vi "myRIO_BRig_RT_dataMTrig_main__wWarmUp.vi"(0 "input_dataMTrig":u16[](array[numeric]), 2 "input_Solenoid_trig_L":bool, 3 "input_Solenoid_trig_R":bool, 4 "input_Audio_trig_L":bool, 5 "input_Audio_trig_R":bool, 7 "input_Laser_trig":bool, 8 "WarmUp":bool) -> (13 "output_Laser":bool, 14 "output_dataMTrig":u16[](array[numeric]), 16 "output_Solenoid_L":bool, 17 "output_Solenoid_R":bool, 18 "output_Audio_L":bool, 19 "output_Audio_R":bool)   [LabVIEW 2014]
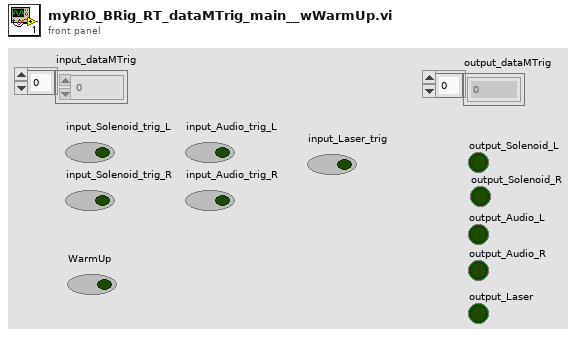
[diagram p1: front panel]
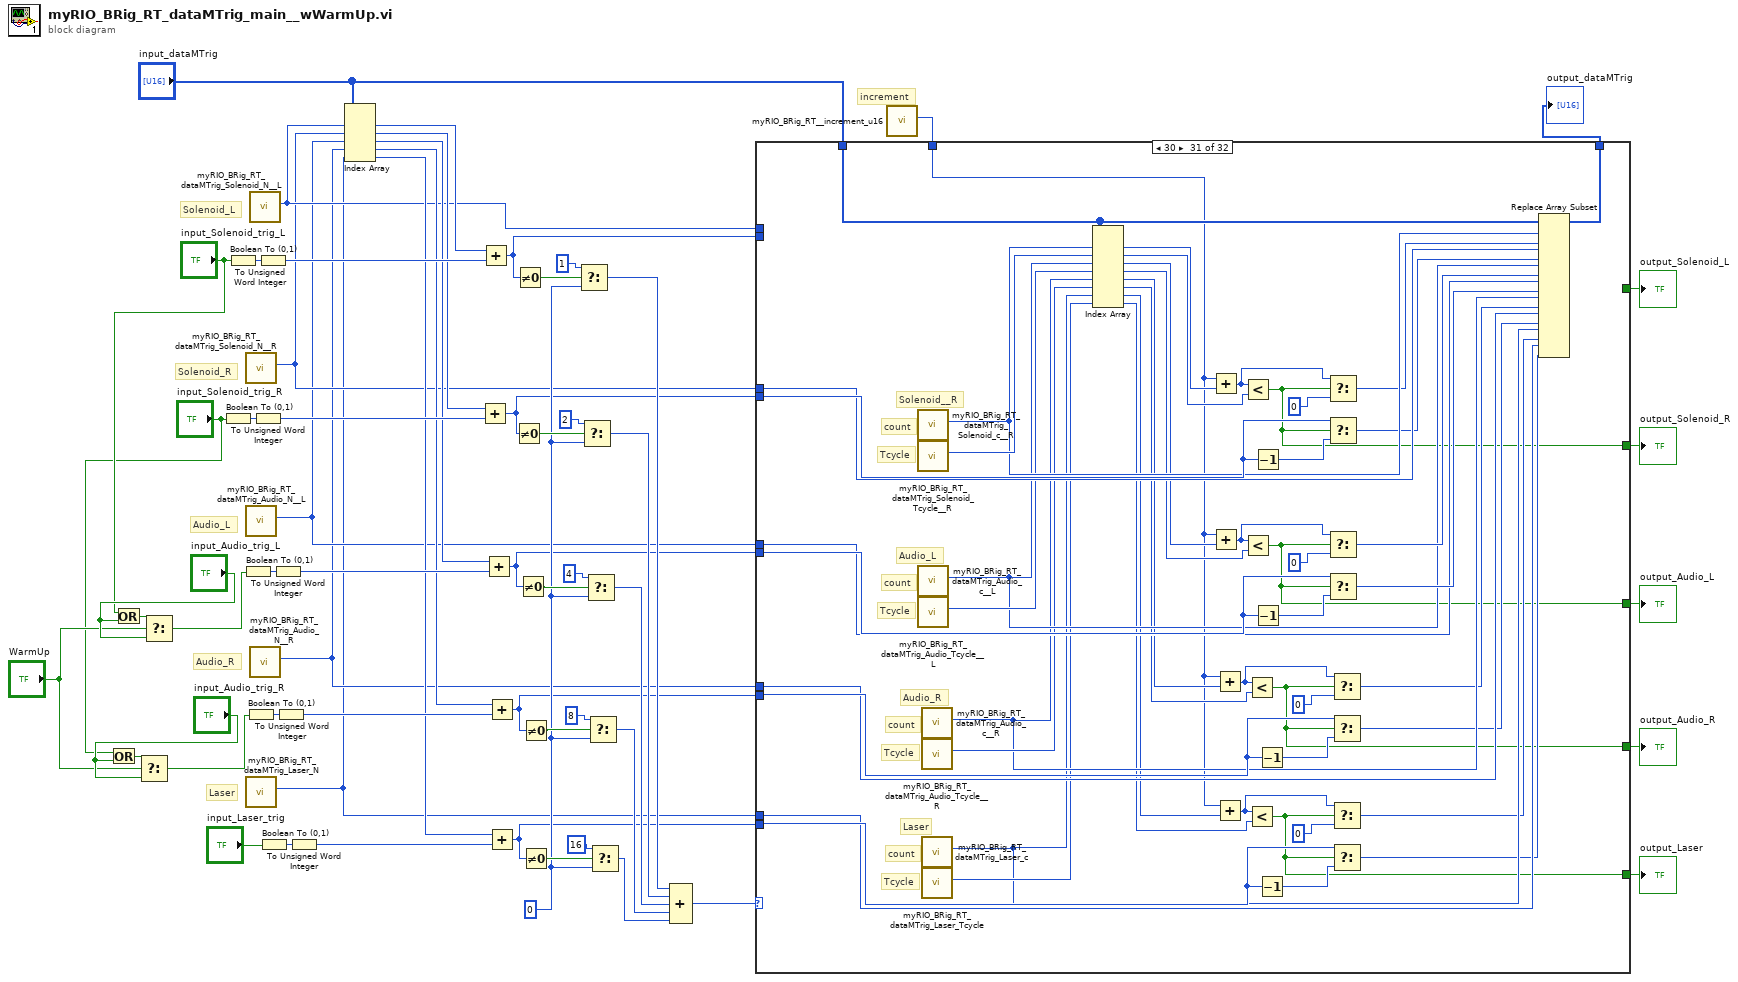
[diagram p0: block diagram]
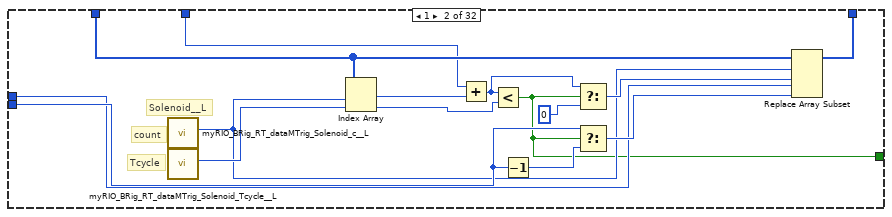
[diagram p3: hidden frame]
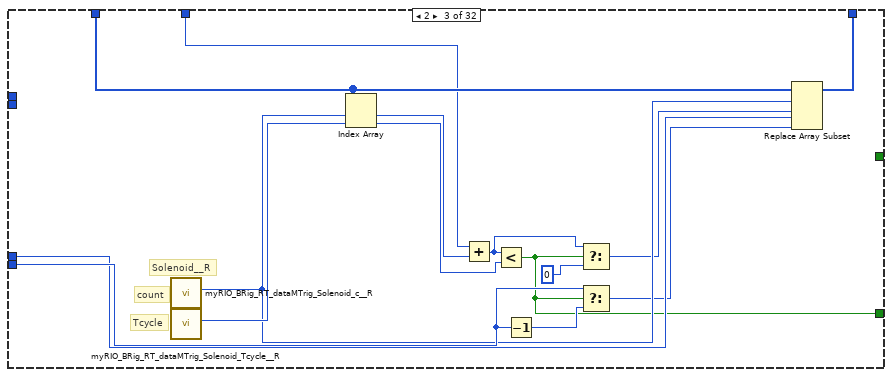
[diagram p4: hidden frame]
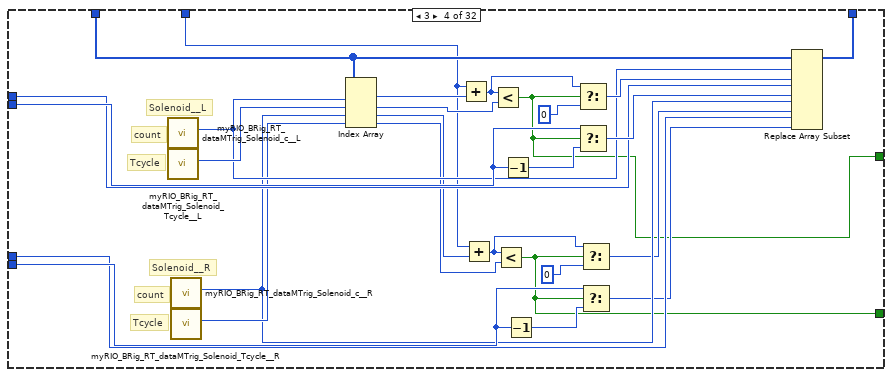
[diagram p5: hidden frame]
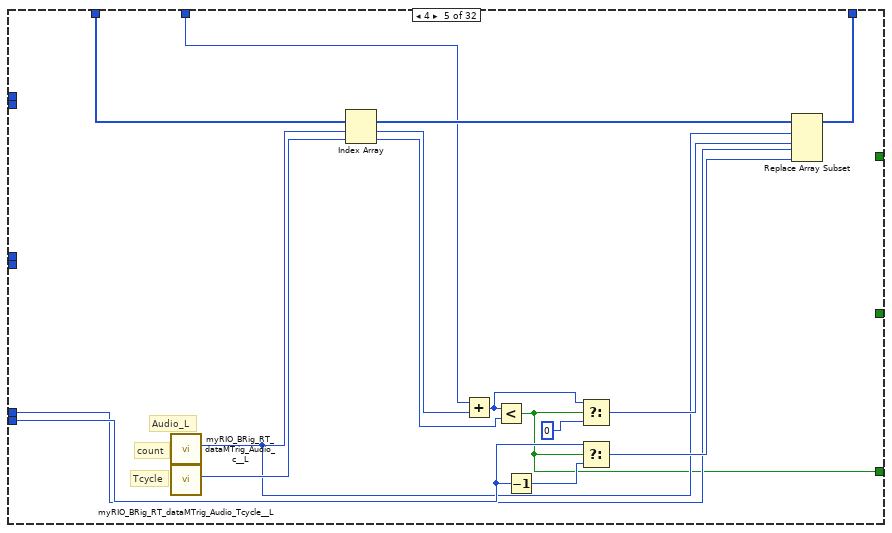
[diagram p6: hidden frame]
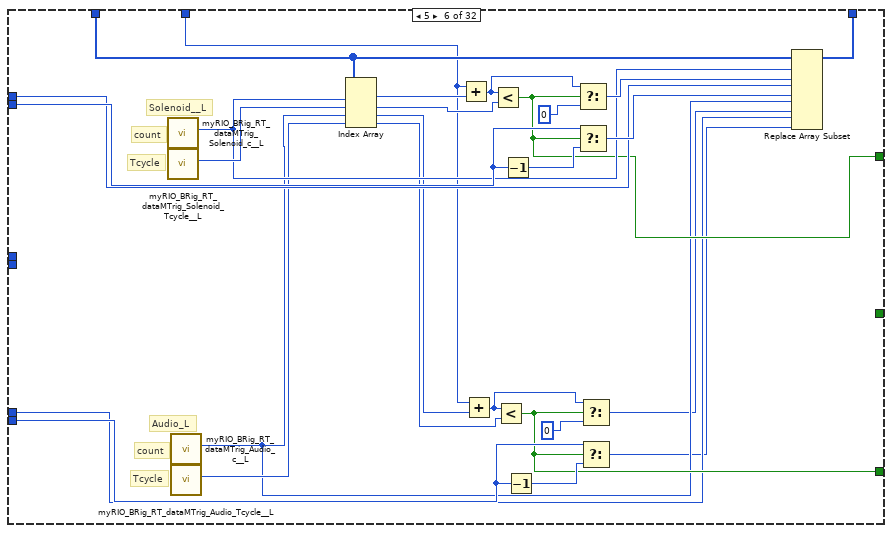
[diagram p7: hidden frame]
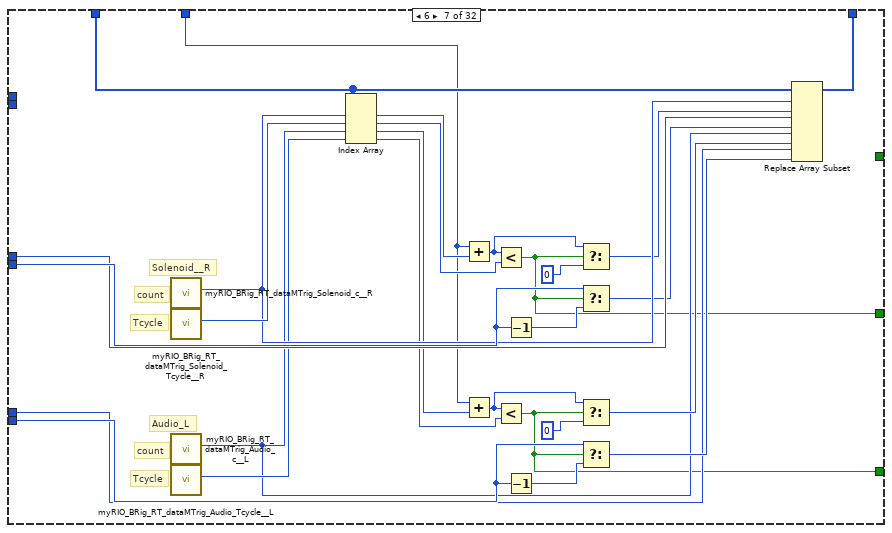
[diagram p8: hidden frame]
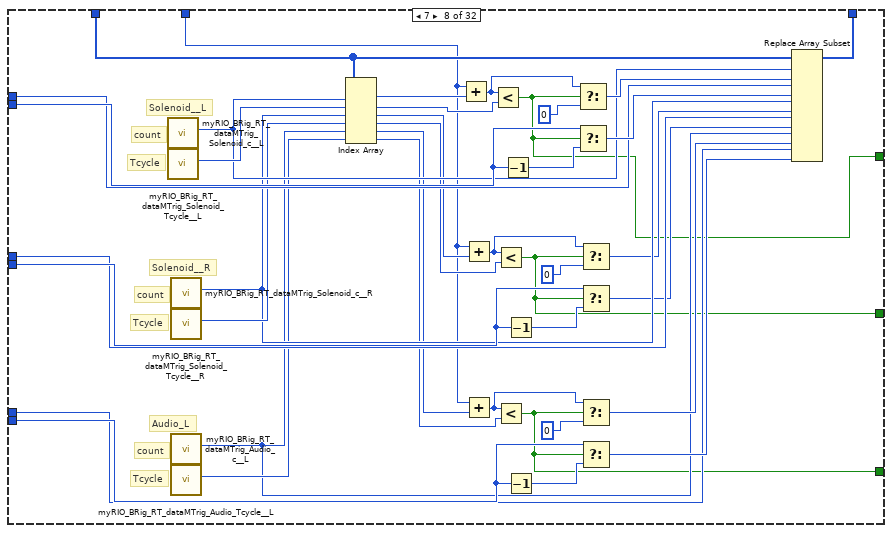
[diagram p9: hidden frame]
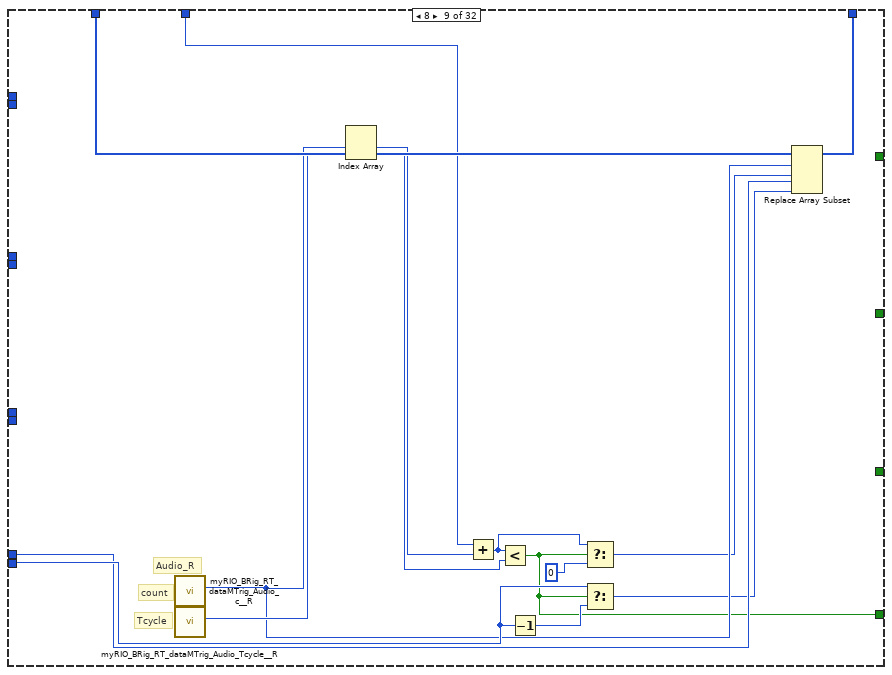
[diagram p10: hidden frame]
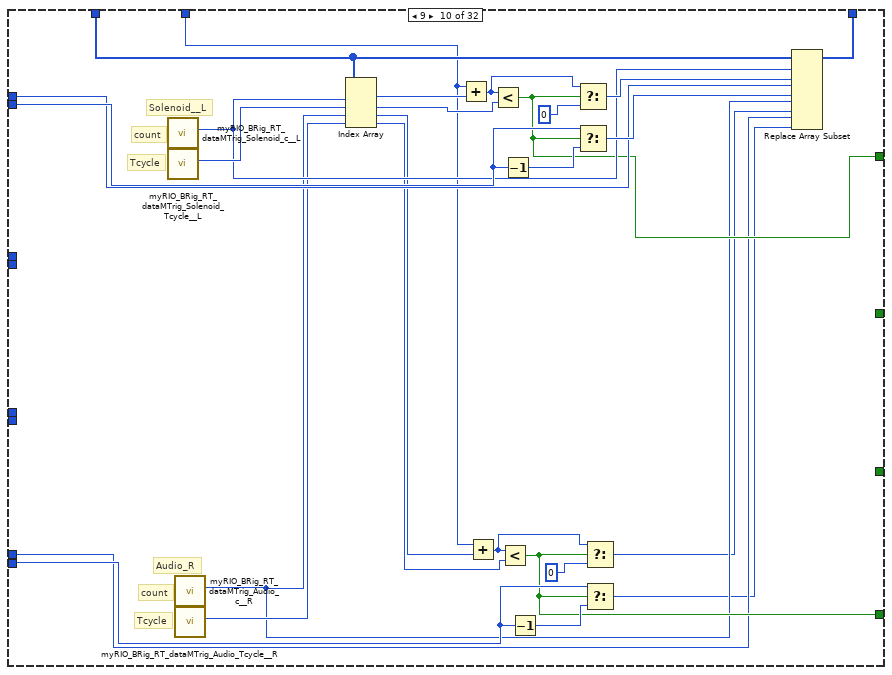
[diagram p11: hidden frame]
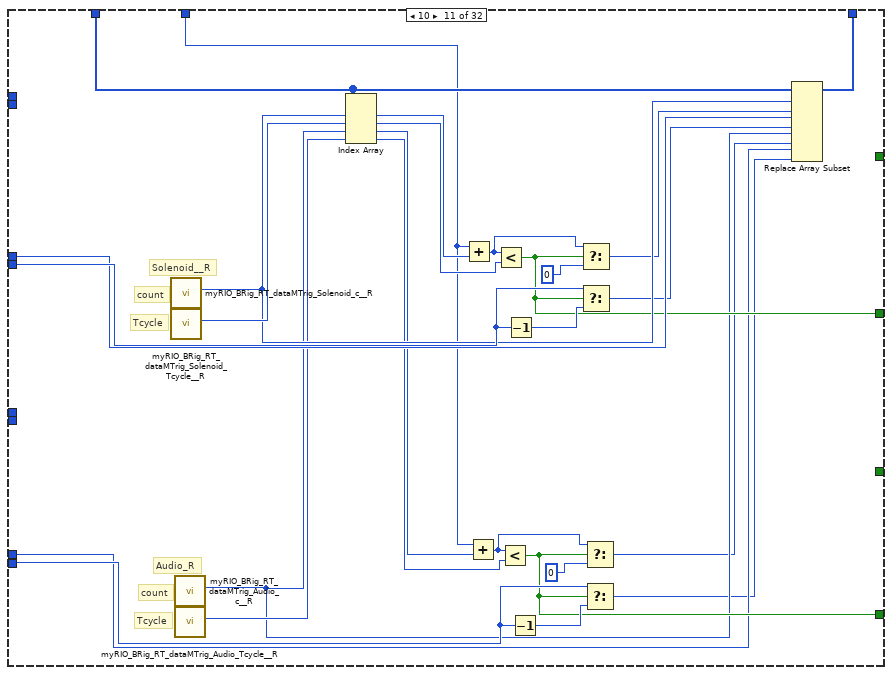
[diagram p12: hidden frame]
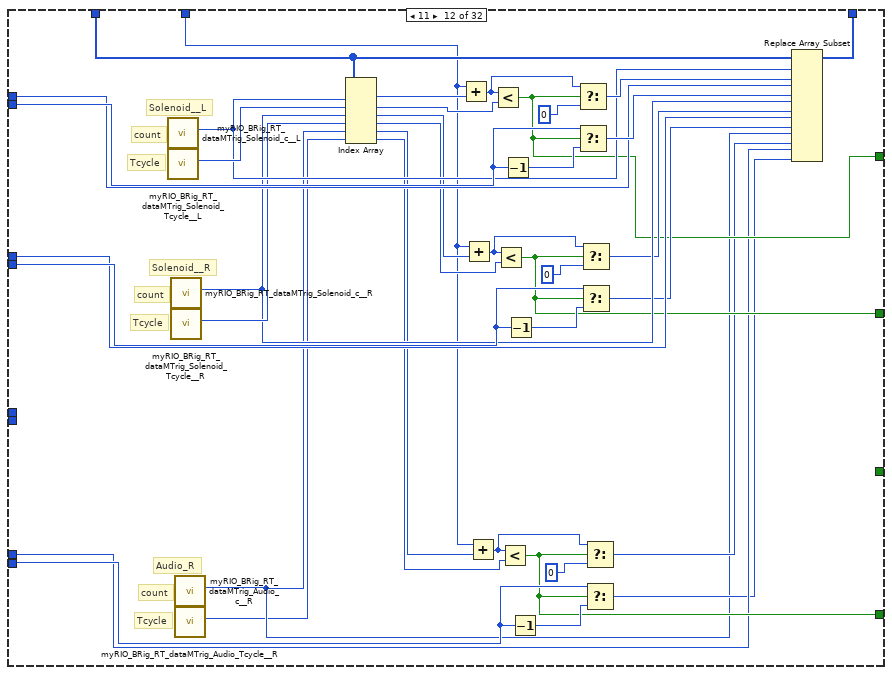
[diagram p13: hidden frame]
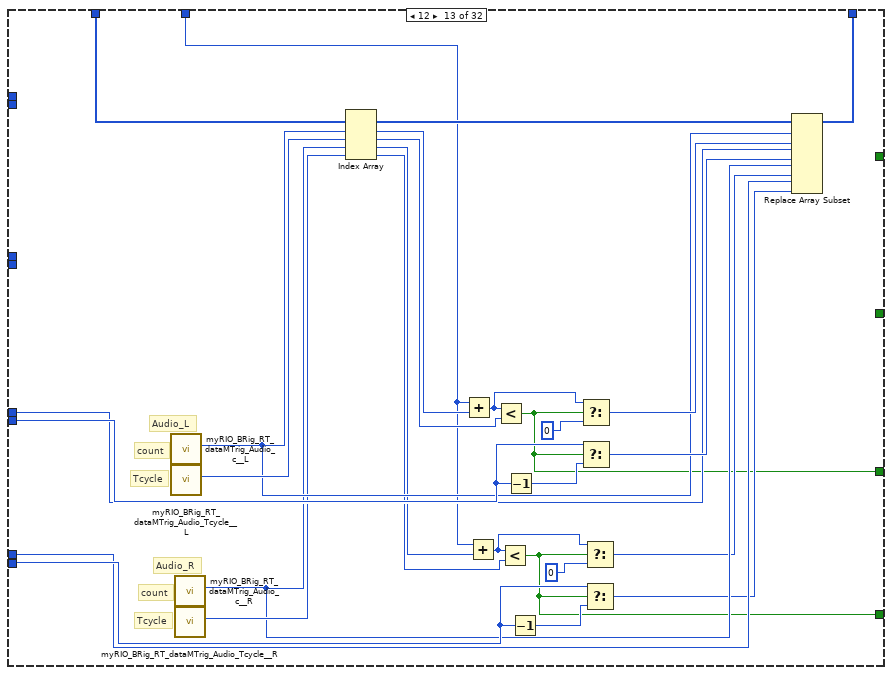
[diagram p14: hidden frame]
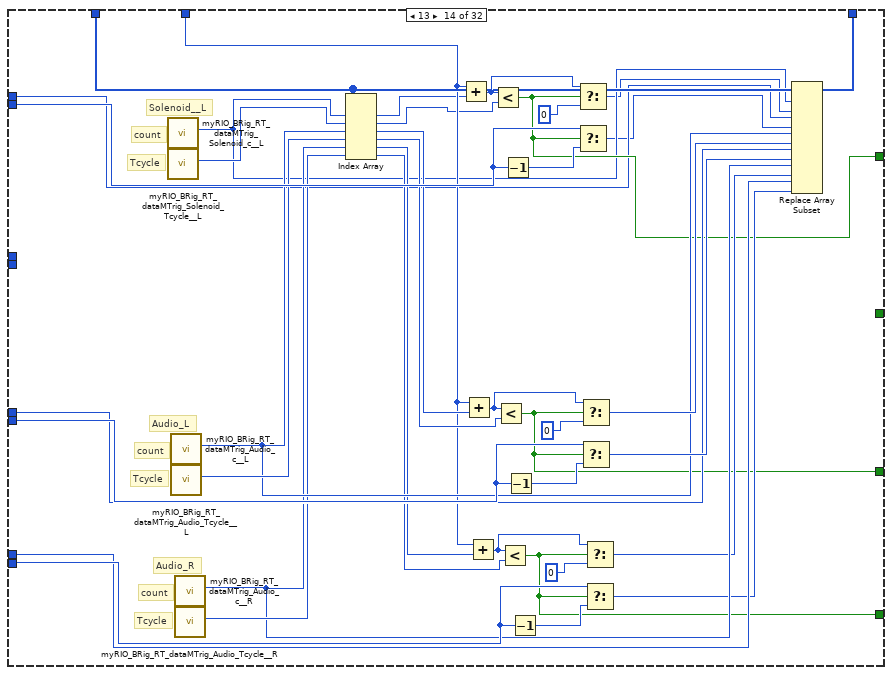
[diagram p15: hidden frame]
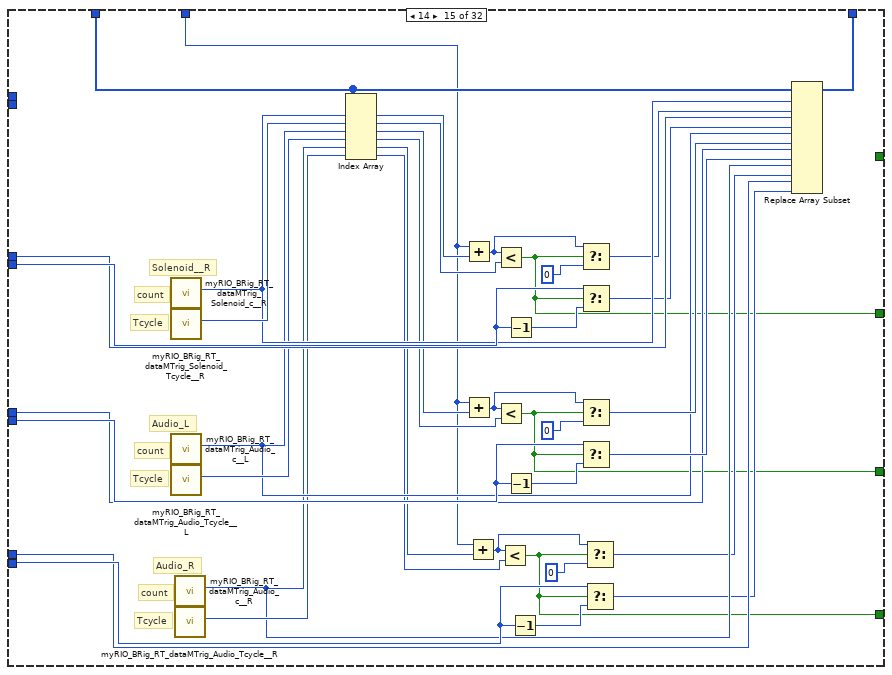
[diagram p16: hidden frame]
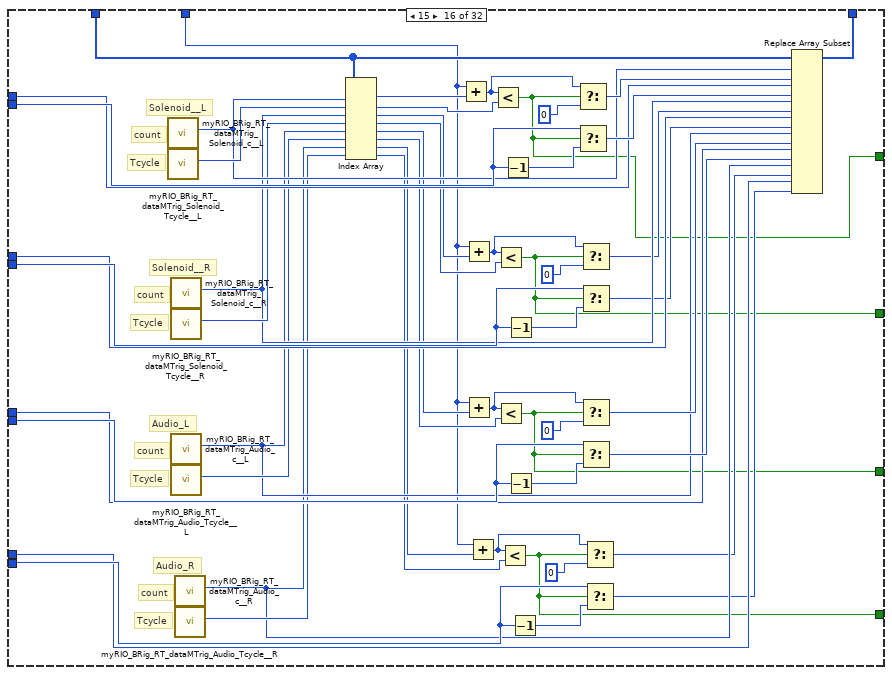
[diagram p17: hidden frame]
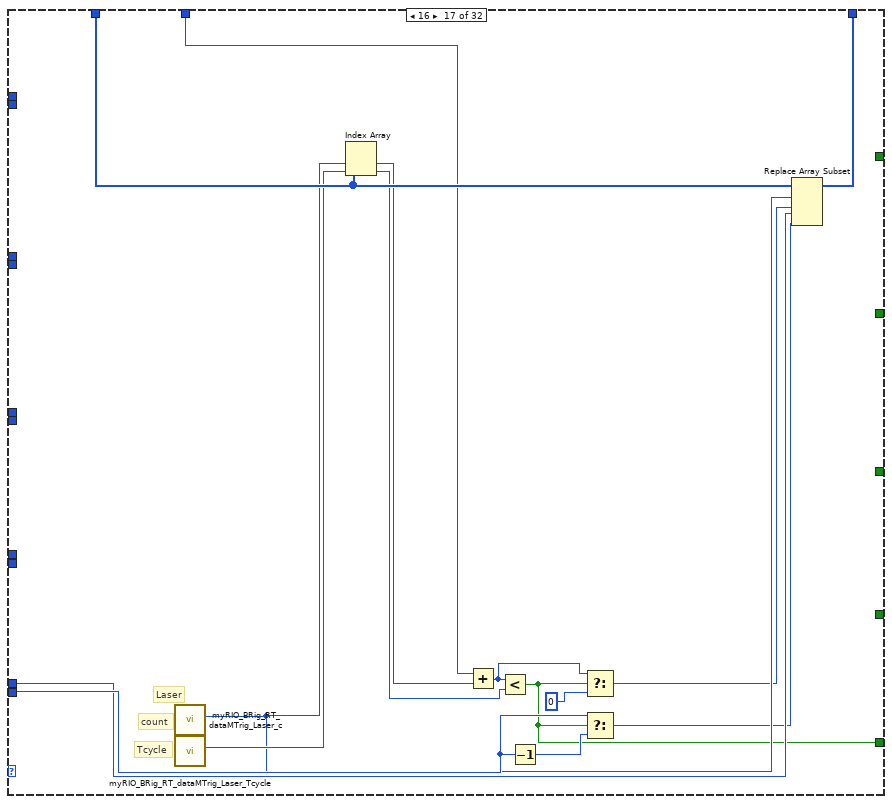
[diagram p18: hidden frame]
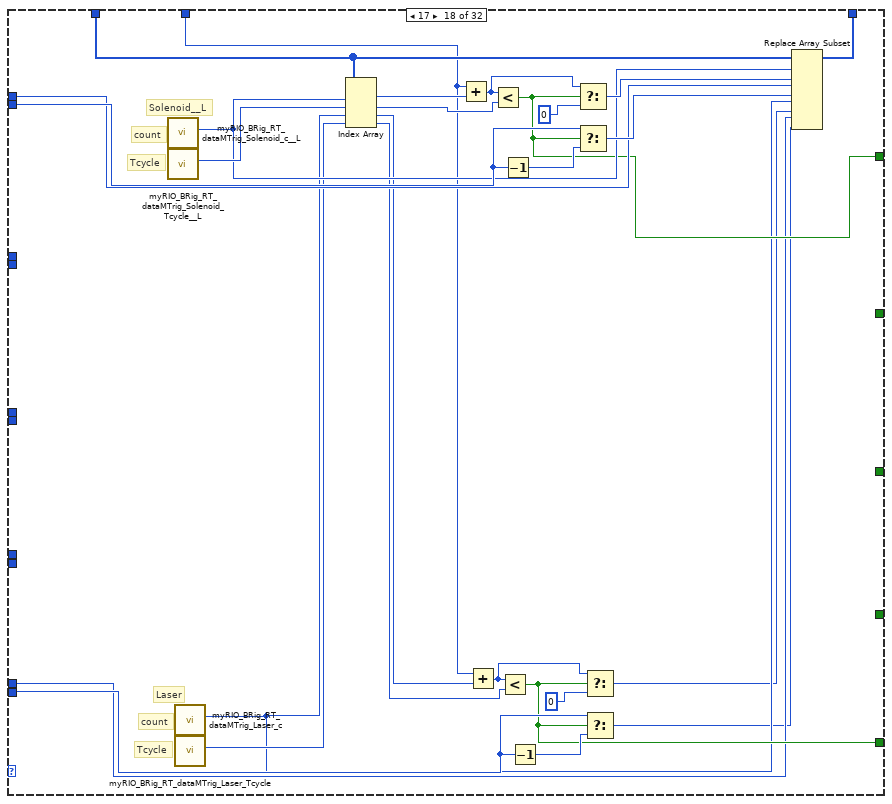
[diagram p19: hidden frame]
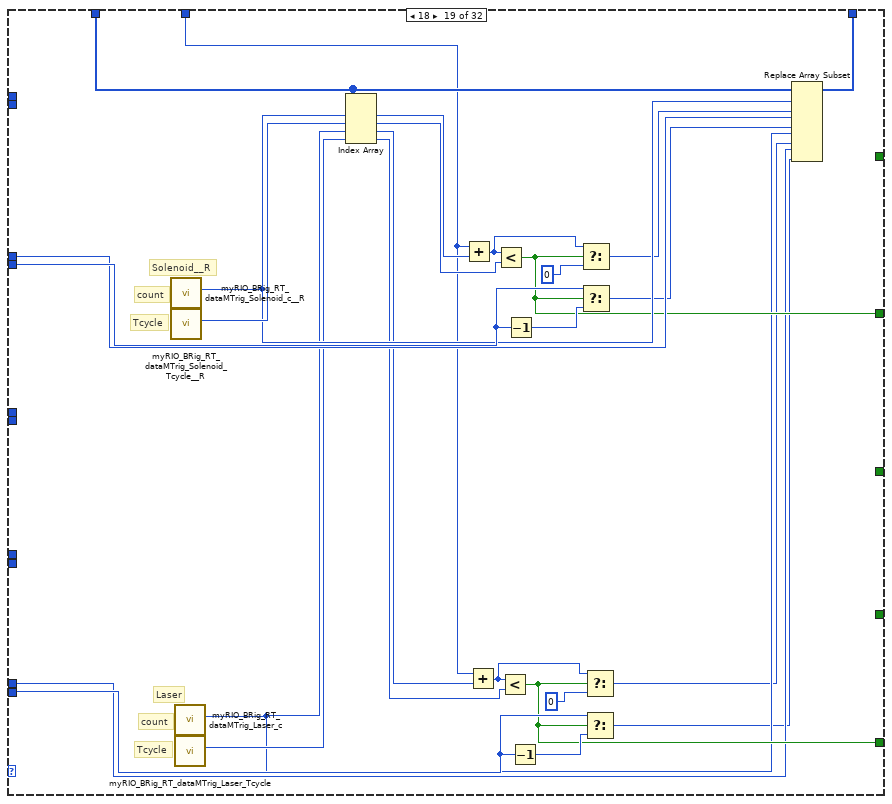
[diagram p20: hidden frame]
diagram:
  w34 = u8 0
  # "increment"
  # "Laser"
  # "Audio_R"
  # "Audio_L"
  # "Solenoid_R"
  # "Solenoid_L"
  n1 = Or(x="input_Solenoid_trig_R", y="input_Audio_trig_R") -> (x .or. y?=w5:bool)
  n2 = Or(x="input_Solenoid_trig_L", y="input_Audio_trig_L") -> (x .or. y?=w8:bool)
  n3 = Select(t=w5, s="WarmUp", f="input_Audio_trig_R") -> (s? t:f=w3:bool)
  n4 = Select(t=w8, s="WarmUp", f="input_Audio_trig_L") -> (s? t:f=w9:bool)
  n5 = Boolean To (0,1)(Boolean="input_Solenoid_trig_R") -> (0, 1=w59:i16)
  n6 = Boolean To (0,1)(Boolean="input_Solenoid_trig_L") -> (0, 1=w60:i16)
  n7 = Boolean To (0,1)(Boolean=w9) -> (0, 1=w58:i16)
  n8 = call "myRIO_BRig_RT_dataMTrig_Solenoid_N__R.vi"() -> ("output_Solenoid_N__R"=w19:i32)  [unwired: 11 in]
  n9 = call "myRIO_BRig_RT_dataMTrig_Audio_N__L.vi"() -> ("output_Audio_N__L"=w17:i32)  [unwired: 11 in]
  n10 = Boolean To (0,1)(Boolean=w3) -> (0, 1=w57:i16)
  n11 = call "myRIO_BRig_RT_dataMTrig_Laser_N.vi"() -> ("output_Laser_c"=w15:i32)  [unwired: 11 in]
  n12 = call "myRIO_BRig_RT_dataMTrig_Solenoid_N__L.vi"() -> ("output_Solenoid_N__L"=w20:i32)  [unwired: 11 in]
  n13 = call "myRIO_BRig_RT_dataMTrig_Audio_N__R.vi"() -> ("output_Audio_N__R"=w16:i32)  [unwired: 11 in]
  n14 = To Unsigned Word Integer(number=w59) -> (unsigned 16bit integer=w52:u16)
  n15 = To Unsigned Word Integer(number=w60) -> (unsigned 16bit integer=w54:u16)
  n16 = Boolean To (0,1)(Boolean="input_Laser_trig") -> (0, 1=w56:i16)
  n17 = To Unsigned Word Integer(number=w58) -> (unsigned 16bit integer=w50:u16)
  n18 = To Unsigned Word Integer(number=w57) -> (unsigned 16bit integer=w48:u16)
  n19 = To Unsigned Word Integer(number=w56) -> (unsigned 16bit integer=w46:u16)
  n20 = Index Array(array="input_dataMTrig", index #1=w20, index #2=w19, index #3=w17, index #4=w16, index #5=w15) -> (element #1=w53:u16, element #2=w51:u16, element #3=w49:u16, element #4=w47:u16, element #5=w45:u16)
  n21 = Add(x=w51, y=w52) -> (x+y=w25:u16)
  n22 = Add(x=w53, y=w54) -> (x+y=w27:u16)
  n23 = Add(x=w49, y=w50) -> (x+y=w24:u16)
  n24 = Add(x=w47, y=w48) -> (x+y=w23:u16)
  n25 = Add(x=w45, y=w46) -> (x+y=w22:u16)
  n26 = Not Equal To 0?(x=w25) -> (x != 0?=w35:bool)
  n27 = Not Equal To 0?(x=w27) -> (x != 0?=w44:bool)
  n28 = Not Equal To 0?(x=w24) -> (x != 0?=w36:bool)
  n29 = Not Equal To 0?(x=w23) -> (x != 0?=w37:bool)
  n30 = Not Equal To 0?(x=w22) -> (x != 0?=w38:bool)
  n31 = Select(t=u8 1, s=w44, f=w34) -> (s? t:f=w29:u8)
  n32 = Select(t=u8 2, s=w35, f=w34) -> (s? t:f=w30:u8)
  n33 = Select(t=u8 4, s=w36, f=w34) -> (s? t:f=w31:u8)
  n34 = Select(t=u8 8, s=w37, f=w34) -> (s? t:f=w32:u8)
  n35 = Select(t=u8 16, s=w38, f=w34) -> (s? t:f=w33:u8)
  n36 = Compound Arithmetic op=ADD(w29, w30, w31, w32, w33) -> (w28:u8)
  n37 = call "myRIO_BRig_RT__increment_u16.vi"() -> ("output_increment__u16"=w21:u16)  [unwired: 11 in]
  n38 = case shown="30" w28 {
    tunnel: w27 -> [_ w67 _ w109 _ w151 _ w217 _ w259 _ w325 _ w396 _ w481 _ w523 _ w589 _ w655 _ w745 _ w816 _ w901 _ w996 _ w1105]
    tunnel: "input_dataMTrig" -> [w61 w70 w91 w112 w133 w154 w187 w220 w241 w262 w295 w328 w361 w397 w439 w484 w505 w526 w559 w592 w625 w658 w703 w748 w781 w817 w859 w904 w949 w997 w1051 w1108]
    tunnel: w25 -> [_ _ w87 w103 _ _ w183 w211 _ _ w291 w319 _ _ w435 w475 _ _ w555 w583 _ _ w699 w739 _ _ w855 w895 _ _ w1047 w1099]
    tunnel: w24 -> [_ _ _ _ w128 w144 w171 w199 _ _ _ _ w356 w391 w423 w463 _ _ _ _ w620 w648 w687 w727 _ _ _ _ w944 w991 w1035 w1087]
    tunnel: w23 -> [_ _ _ _ _ _ _ _ w236 w252 w279 w307 w345 w380 w412 w452 _ _ _ _ _ _ _ _ w776 w811 w850 w883 w933 w980 w1024 w1076]
    tunnel: w22 -> [_ _ _ _ _ _ _ _ _ _ _ _ _ _ _ _ w500 w516 w543 w571 w609 w644 w676 w716 w765 w800 w839 w879 w922 w969 w1013 w1065]
    tunnel: w21 -> [_ w63 w78 w94 w120 w143 w163 w191 w228 w251 w278 w306 w337 w372 w404 w444 w499 w515 w542 w570 w608 w643 w675 w715 w764 w799 w838 w878 w921 w968 w1012 w1064]
    tunnel: w20 -> [_ w66 _ w108 _ w150 _ w216 _ w258 _ w324 _ w363 _ w480 _ w522 _ w588 _ w654 _ w744 _ w783 _ w900 _ w951 _ w1104]
    tunnel: w19 -> [_ _ w81 w97 _ _ w177 w205 _ _ w285 w313 _ _ w429 w469 _ _ w549 w577 _ _ w693 w733 _ _ w826 w889 _ _ w1041 w1093]
    tunnel: [w61 w64 w79 w95 w132 w148 w175 w203 w240 w256 w283 w311 w360 w395 w427 w467 w504 w520 w547 w575 w624 w652 w691 w731 w780 w815 w854 w887 w948 w995 w1039 w1091] -> w18
    tunnel: w17 -> [_ _ _ _ w122 w135 w165 w193 _ _ _ _ w350 w385 w417 w457 _ _ _ _ w614 w631 w681 w721 _ _ _ _ w938 w985 w1029 w1081]
    tunnel: w16 -> [_ _ _ _ _ _ _ _ w231 w243 w270 w301 w340 w375 w407 w447 _ _ _ _ _ _ _ _ w771 w806 w845 w865 w928 w975 w1019 w1071]
    tunnel: w15 -> [_ _ _ _ _ _ _ _ _ _ _ _ _ _ _ _ w494 w507 w534 w561 w600 w627 w666 w705 w759 w794 w833 w861 w916 w963 w1007 w1059]
    tunnel: [_ _ _ _ _ _ _ _ _ _ _ _ _ _ _ _ w491 w514 w541 w569 w607 w642 w674 w714 w756 w791 w830 w877 w913 w960 w1004 w1056] -> w10
    tunnel: [_ _ _ _ _ _ _ _ w227 w250 w277 w305 w336 w371 w403 w443 _ _ _ _ _ _ _ _ w755 w790 w829 w876 w912 w959 w1003 w1055] -> w11
    tunnel: [_ _ _ _ w119 w142 w162 w190 _ _ _ _ w335 w370 w402 w442 _ _ _ _ w606 w641 w673 w713 _ _ _ _ w911 w958 w1002 w1054] -> w12
    tunnel: [_ _ w77 w93 _ _ w161 w189 _ _ w276 w304 _ _ w401 w441 _ _ w540 w568 _ _ w672 w712 _ _ w828 w875 _ _ w1001 w1053] -> w13
    tunnel: [_ w62 _ w92 _ w141 _ w188 _ w249 _ w303 _ w369 _ w440 _ w513 _ w567 _ w640 _ w711 _ w789 _ w874 _ w957 _ w1052] -> w14
    frame 0, Default {
    }
    frame 1 {
      # "Solenoid__L"
      # "Tcycle"
      # "count"
      n39 = call "myRIO_BRig_RT_dataMTrig_Solenoid_c__L.vi"() -> ("output_Solenoid_c__L"=w65:i32)  [unwired: 11 in]
      n40 = call "myRIO_BRig_RT_dataMTrig_Solenoid_Tcycle__L.vi"() -> ("output_Solenoid_Tcycle__L"=w76:i32)  [unwired: 11 in]
      n41 = Index Array(array=w70, index #1=w65, index #2=w76) -> (element #1=w75:u16, element #2=w74:u16)
      n42 = Add(x=w63, y=w75) -> (x+y=w72:u16)
      n43 = Less?(x=w72, y=w74) -> (x < y?=w62:bool)
      n44 = Decrement(x=w67) -> (x-1=w73:u16)
      n45 = Select(t=w72, s=w62, f=u16 0) -> (s? t:f=w68:u16)
      n46 = Select(t=w67, s=w62, f=w73) -> (s? t:f=w69:u16)
      n47 = Replace Array Subset(array=w70, new element #1=w68, index #1=w65, new element #2=w69, index #2=w66) -> (w64:u16[])
    }
    frame 2 {
      # "Solenoid__R"
      # "Tcycle"
      # "count"
      n48 = call "myRIO_BRig_RT_dataMTrig_Solenoid_c__R.vi"() -> ("output_Solenoid_c__R"=w83:i32)  [unwired: 11 in]
      n49 = call "myRIO_BRig_RT_dataMTrig_Solenoid_Tcycle__R.vi"() -> ("output_Solenoid_Tcycle__R"=w86:i32)  [unwired: 11 in]
      n50 = Index Array(array=w91, index #1=w83, index #2=w86) -> (element #1=w85:u16, element #2=w84:u16)
      n51 = Add(x=w78, y=w85) -> (x+y=w89:u16)
      n52 = Less?(x=w89, y=w84) -> (x < y?=w77:bool)
      n53 = Decrement(x=w87) -> (x-1=w90:u16)
      n54 = Select(t=w89, s=w77, f=u16 0) -> (s? t:f=w82:u16)
      n55 = Select(t=w87, s=w77, f=w90) -> (s? t:f=w80:u16)
      n56 = Replace Array Subset(array=w91, new element #1=w82, index #1=w83, new element #2=w80, index #2=w81) -> (w79:u16[])
    }
    frame 3 {
      # "Solenoid__R"
      # "Tcycle"
      # "count"
      # "Solenoid__L"
      # "Tcycle"
      # "count"
      n57 = call "myRIO_BRig_RT_dataMTrig_Solenoid_c__L.vi"() -> ("output_Solenoid_c__L"=w107:i32)  [unwired: 11 in]
      n58 = call "myRIO_BRig_RT_dataMTrig_Solenoid_Tcycle__L.vi"() -> ("output_Solenoid_Tcycle__L"=w118:i32)  [unwired: 11 in]
      n59 = call "myRIO_BRig_RT_dataMTrig_Solenoid_c__R.vi"() -> ("output_Solenoid_c__R"=w99:i32)  [unwired: 11 in]
      n60 = call "myRIO_BRig_RT_dataMTrig_Solenoid_Tcycle__R.vi"() -> ("output_Solenoid_Tcycle__R"=w102:i32)  [unwired: 11 in]
      n61 = Index Array(array=w112, index #1=w107, index #2=w118, index #3=w99, index #4=w102) -> (element #1=w117:u16, element #2=w116:u16, element #3=w101:u16, element #4=w100:u16)
      n62 = Add(x=w94, y=w117) -> (x+y=w114:u16)
      n63 = Add(x=w94, y=w101) -> (x+y=w105:u16)
      n64 = Less?(x=w114, y=w116) -> (x < y?=w92:bool)
      n65 = Less?(x=w105, y=w100) -> (x < y?=w93:bool)
      n66 = Decrement(x=w109) -> (x-1=w115:u16)
      n67 = Decrement(x=w103) -> (x-1=w106:u16)
      n68 = Select(t=w114, s=w92, f=u16 0) -> (s? t:f=w110:u16)
      n69 = Select(t=w109, s=w92, f=w115) -> (s? t:f=w111:u16)
      n70 = Select(t=w105, s=w93, f=u16 0) -> (s? t:f=w98:u16)
      n71 = Select(t=w103, s=w93, f=w106) -> (s? t:f=w96:u16)
      n72 = Replace Array Subset(array=w112, new element #1=w110, index #1=w107, new element #2=w111, index #2=w108, new element #3=w98, index #3=w99, new element #4=w96, index #4=w97) -> (w95:u16[])
    }
    frame 4 {
      # "Audio_L"
      # "Tcycle"
      # "count"
      n73 = call "myRIO_BRig_RT_dataMTrig_Audio_c__L.vi"() -> ("output_Audio_c__L"=w121:i32)  [unwired: 11 in]
      n74 = call "myRIO_BRig_RT_dataMTrig_Audio_Tcycle__L.vi"() -> ("output_Audio_Tcycle__L"=w127:i32)  [unwired: 11 in]
      n75 = Index Array(array=w133, index #1=w121, index #2=w127) -> (element #1=w126:u16, element #2=w125:u16)
      n76 = Add(x=w120, y=w126) -> (x+y=w130:u16)
      n77 = Less?(x=w130, y=w125) -> (x < y?=w119:bool)
      n78 = Decrement(x=w128) -> (x-1=w131:u16)
      n79 = Select(t=w130, s=w119, f=u16 0) -> (s? t:f=w124:u16)
      n80 = Select(t=w128, s=w119, f=w131) -> (s? t:f=w123:u16)
      n81 = Replace Array Subset(array=w133, new element #1=w124, index #1=w121, new element #2=w123, index #2=w122) -> (w132:u16[])
    }
    frame 5 {
      # "Audio_L"
      # "Tcycle"
      # "count"
      # "Solenoid__L"
      # "Tcycle"
      # "count"
      n82 = call "myRIO_BRig_RT_dataMTrig_Solenoid_c__L.vi"() -> ("output_Solenoid_c__L"=w149:i32)  [unwired: 11 in]
      n83 = call "myRIO_BRig_RT_dataMTrig_Solenoid_Tcycle__L.vi"() -> ("output_Solenoid_Tcycle__L"=w160:i32)  [unwired: 11 in]
      n84 = call "myRIO_BRig_RT_dataMTrig_Audio_c__L.vi"() -> ("output_Audio_c__L"=w137:i32)  [unwired: 11 in]
      n85 = call "myRIO_BRig_RT_dataMTrig_Audio_Tcycle__L.vi"() -> ("output_Audio_Tcycle__L"=w140:i32)  [unwired: 11 in]
      n86 = Index Array(array=w154, index #1=w149, index #2=w160, index #3=w137, index #4=w140) -> (element #1=w159:u16, element #2=w158:u16, element #3=w139:u16, element #4=w138:u16)
      n87 = Add(x=w143, y=w159) -> (x+y=w156:u16)
      n88 = Add(x=w143, y=w139) -> (x+y=w146:u16)
      n89 = Less?(x=w156, y=w158) -> (x < y?=w141:bool)
      n90 = Less?(x=w146, y=w138) -> (x < y?=w142:bool)
      n91 = Decrement(x=w151) -> (x-1=w157:u16)
      n92 = Decrement(x=w144) -> (x-1=w147:u16)
      n93 = Select(t=w156, s=w141, f=u16 0) -> (s? t:f=w152:u16)
      n94 = Select(t=w151, s=w141, f=w157) -> (s? t:f=w153:u16)
      n95 = Select(t=w146, s=w142, f=u16 0) -> (s? t:f=w136:u16)
      n96 = Select(t=w144, s=w142, f=w147) -> (s? t:f=w134:u16)
      n97 = Replace Array Subset(array=w154, new element #1=w152, index #1=w149, new element #2=w153, index #2=w150, new element #3=w136, index #3=w137, new element #4=w134, index #4=w135) -> (w148:u16[])
    }
    frame 6 {
      # "Audio_L"
      # "Tcycle"
      # "count"
      # "Solenoid__R"
      # "Tcycle"
      # "count"
      n98 = call "myRIO_BRig_RT_dataMTrig_Solenoid_c__R.vi"() -> ("output_Solenoid_c__R"=w179:i32)  [unwired: 11 in]
      n99 = call "myRIO_BRig_RT_dataMTrig_Solenoid_Tcycle__R.vi"() -> ("output_Solenoid_Tcycle__R"=w182:i32)  [unwired: 11 in]
      n100 = call "myRIO_BRig_RT_dataMTrig_Audio_c__L.vi"() -> ("output_Audio_c__L"=w164:i32)  [unwired: 11 in]
      n101 = call "myRIO_BRig_RT_dataMTrig_Audio_Tcycle__L.vi"() -> ("output_Audio_Tcycle__L"=w170:i32)  [unwired: 11 in]
      n102 = Index Array(array=w187, index #1=w179, index #2=w182, index #3=w164, index #4=w170) -> (element #1=w181:u16, element #2=w180:u16, element #3=w169:u16, element #4=w168:u16)
      n103 = Add(x=w163, y=w181) -> (x+y=w185:u16)
      n104 = Add(x=w163, y=w169) -> (x+y=w173:u16)
      n105 = Less?(x=w185, y=w180) -> (x < y?=w161:bool)
      n106 = Less?(x=w173, y=w168) -> (x < y?=w162:bool)
      n107 = Decrement(x=w183) -> (x-1=w186:u16)
      n108 = Decrement(x=w171) -> (x-1=w174:u16)
      n109 = Select(t=w185, s=w161, f=u16 0) -> (s? t:f=w178:u16)
      n110 = Select(t=w183, s=w161, f=w186) -> (s? t:f=w176:u16)
      n111 = Select(t=w173, s=w162, f=u16 0) -> (s? t:f=w167:u16)
      n112 = Select(t=w171, s=w162, f=w174) -> (s? t:f=w166:u16)
      n113 = Replace Array Subset(array=w187, new element #1=w178, index #1=w179, new element #2=w176, index #2=w177, new element #3=w167, index #3=w164, new element #4=w166, index #4=w165) -> (w175:u16[])
    }
    frame 7 {
      # "Audio_L"
      # "Tcycle"
      # "count"
      # "Solenoid__R"
      # "Tcycle"
      # "count"
      # "Solenoid__L"
      # "Tcycle"
      # "count"
      n114 = call "myRIO_BRig_RT_dataMTrig_Solenoid_c__L.vi"() -> ("output_Solenoid_c__L"=w215:i32)  [unwired: 11 in]
      n115 = call "myRIO_BRig_RT_dataMTrig_Solenoid_Tcycle__L.vi"() -> ("output_Solenoid_Tcycle__L"=w226:i32)  [unwired: 11 in]
      n116 = call "myRIO_BRig_RT_dataMTrig_Solenoid_c__R.vi"() -> ("output_Solenoid_c__R"=w207:i32)  [unwired: 11 in]
      n117 = call "myRIO_BRig_RT_dataMTrig_Solenoid_Tcycle__R.vi"() -> ("output_Solenoid_Tcycle__R"=w210:i32)  [unwired: 11 in]
      n118 = call "myRIO_BRig_RT_dataMTrig_Audio_c__L.vi"() -> ("output_Audio_c__L"=w192:i32)  [unwired: 11 in]
      n119 = call "myRIO_BRig_RT_dataMTrig_Audio_Tcycle__L.vi"() -> ("output_Audio_Tcycle__L"=w198:i32)  [unwired: 11 in]
      n120 = Index Array(array=w220, index #1=w215, index #2=w226, index #3=w207, index #4=w210, index #5=w192, index #6=w198) -> (element #1=w225:u16, element #2=w224:u16, element #3=w209:u16, element #4=w208:u16, element #5=w197:u16, element #6=w196:u16)
      n121 = Add(x=w191, y=w225) -> (x+y=w222:u16)
      n122 = Add(x=w191, y=w209) -> (x+y=w213:u16)
      n123 = Add(x=w191, y=w197) -> (x+y=w201:u16)
      n124 = Less?(x=w222, y=w224) -> (x < y?=w188:bool)
      n125 = Less?(x=w213, y=w208) -> (x < y?=w189:bool)
      n126 = Less?(x=w201, y=w196) -> (x < y?=w190:bool)
      n127 = Decrement(x=w217) -> (x-1=w223:u16)
      n128 = Decrement(x=w211) -> (x-1=w214:u16)
      n129 = Decrement(x=w199) -> (x-1=w202:u16)
      n130 = Select(t=w222, s=w188, f=u16 0) -> (s? t:f=w218:u16)
      n131 = Select(t=w217, s=w188, f=w223) -> (s? t:f=w219:u16)
      n132 = Select(t=w213, s=w189, f=u16 0) -> (s? t:f=w206:u16)
      n133 = Select(t=w211, s=w189, f=w214) -> (s? t:f=w204:u16)
      n134 = Select(t=w201, s=w190, f=u16 0) -> (s? t:f=w195:u16)
      n135 = Select(t=w199, s=w190, f=w202) -> (s? t:f=w194:u16)
      n136 = Replace Array Subset(array=w220, new element #1=w218, index #1=w215, new element #2=w219, index #2=w216, new element #3=w206, index #3=w207, new element #4=w204, index #4=w205, new element #5=w195, index #5=w192, new element #6=w194, index #6=w193) -> (w203:u16[])
    }
    frame 8 {
      # "Audio_R"
      # "Tcycle"
      # "count"
      n137 = call "myRIO_BRig_RT_dataMTrig_Audio_c__R.vi"() -> ("output_Audio_c__R"=w232:i32)  [unwired: 11 in]
      n138 = call "myRIO_BRig_RT_dataMTrig_Audio_Tcycle__R.vi"() -> ("output_Audio_Tcycle__R"=w233:i32)  [unwired: 11 in]
      n139 = Index Array(array=w241, index #1=w232, index #2=w233) -> (element #1=w235:u16, element #2=w234:u16)
      n140 = Add(x=w228, y=w235) -> (x+y=w238:u16)
      n141 = Less?(x=w238, y=w234) -> (x < y?=w227:bool)
      n142 = Decrement(x=w236) -> (x-1=w239:u16)
      n143 = Select(t=w238, s=w227, f=u16 0) -> (s? t:f=w230:u16)
      n144 = Select(t=w236, s=w227, f=w239) -> (s? t:f=w229:u16)
      n145 = Replace Array Subset(array=w241, new element #1=w230, index #1=w232, new element #2=w229, index #2=w231) -> (w240:u16[])
    }
    frame 9 {
      # "Audio_R"
      # "Tcycle"
      # "count"
      # "Solenoid__L"
      # "Tcycle"
      # "count"
      n146 = call "myRIO_BRig_RT_dataMTrig_Solenoid_c__L.vi"() -> ("output_Solenoid_c__L"=w257:i32)  [unwired: 11 in]
      n147 = call "myRIO_BRig_RT_dataMTrig_Solenoid_Tcycle__L.vi"() -> ("output_Solenoid_Tcycle__L"=w268:i32)  [unwired: 11 in]
      n148 = call "myRIO_BRig_RT_dataMTrig_Audio_c__R.vi"() -> ("output_Audio_c__R"=w245:i32)  [unwired: 11 in]
      n149 = call "myRIO_BRig_RT_dataMTrig_Audio_Tcycle__R.vi"() -> ("output_Audio_Tcycle__R"=w248:i32)  [unwired: 11 in]
      n150 = Index Array(array=w262, index #1=w257, index #2=w268, index #3=w245, index #4=w248) -> (element #1=w267:u16, element #2=w266:u16, element #3=w247:u16, element #4=w246:u16)
      n151 = Add(x=w251, y=w267) -> (x+y=w264:u16)
      n152 = Add(x=w251, y=w247) -> (x+y=w254:u16)
      n153 = Less?(x=w264, y=w266) -> (x < y?=w249:bool)
      n154 = Less?(x=w254, y=w246) -> (x < y?=w250:bool)
      n155 = Decrement(x=w259) -> (x-1=w265:u16)
      n156 = Decrement(x=w252) -> (x-1=w255:u16)
      n157 = Select(t=w264, s=w249, f=u16 0) -> (s? t:f=w260:u16)
      n158 = Select(t=w259, s=w249, f=w265) -> (s? t:f=w261:u16)
      n159 = Select(t=w254, s=w250, f=u16 0) -> (s? t:f=w244:u16)
      n160 = Select(t=w252, s=w250, f=w255) -> (s? t:f=w242:u16)
      n161 = Replace Array Subset(array=w262, new element #1=w260, index #1=w257, new element #2=w261, index #2=w258, new element #3=w244, index #3=w245, new element #4=w242, index #4=w243) -> (w256:u16[])
    }
    frame 10 {
      # "Audio_R"
      # "Tcycle"
      # "count"
      # "Solenoid__R"
      # "Tcycle"
      # "count"
      n162 = call "myRIO_BRig_RT_dataMTrig_Solenoid_c__R.vi"() -> ("output_Solenoid_c__R"=w287:i32)  [unwired: 11 in]
      n163 = call "myRIO_BRig_RT_dataMTrig_Solenoid_Tcycle__R.vi"() -> ("output_Solenoid_Tcycle__R"=w290:i32)  [unwired: 11 in]
      n164 = call "myRIO_BRig_RT_dataMTrig_Audio_c__R.vi"() -> ("output_Audio_c__R"=w272:i32)  [unwired: 11 in]
      n165 = call "myRIO_BRig_RT_dataMTrig_Audio_Tcycle__R.vi"() -> ("output_Audio_Tcycle__R"=w275:i32)  [unwired: 11 in]
      n166 = Index Array(array=w295, index #1=w287, index #2=w290, index #3=w272, index #4=w275) -> (element #1=w289:u16, element #2=w288:u16, element #3=w274:u16, element #4=w273:u16)
      n167 = Add(x=w278, y=w289) -> (x+y=w293:u16)
      n168 = Add(x=w278, y=w274) -> (x+y=w281:u16)
      n169 = Less?(x=w293, y=w288) -> (x < y?=w276:bool)
      n170 = Less?(x=w281, y=w273) -> (x < y?=w277:bool)
      n171 = Decrement(x=w291) -> (x-1=w294:u16)
      n172 = Decrement(x=w279) -> (x-1=w282:u16)
      n173 = Select(t=w293, s=w276, f=u16 0) -> (s? t:f=w286:u16)
      n174 = Select(t=w291, s=w276, f=w294) -> (s? t:f=w284:u16)
      n175 = Select(t=w281, s=w277, f=u16 0) -> (s? t:f=w271:u16)
      n176 = Select(t=w279, s=w277, f=w282) -> (s? t:f=w269:u16)
      n177 = Replace Array Subset(array=w295, new element #1=w286, index #1=w287, new element #2=w284, index #2=w285, new element #3=w271, index #3=w272, new element #4=w269, index #4=w270) -> (w283:u16[])
    }
    frame 11 {
      # "Audio_R"
      # "Tcycle"
      # "count"
      # "Solenoid__R"
      # "Tcycle"
      # "count"
      # "Solenoid__L"
      # "Tcycle"
      # "count"
      n178 = call "myRIO_BRig_RT_dataMTrig_Solenoid_c__L.vi"() -> ("output_Solenoid_c__L"=w323:i32)  [unwired: 11 in]
      n179 = call "myRIO_BRig_RT_dataMTrig_Solenoid_Tcycle__L.vi"() -> ("output_Solenoid_Tcycle__L"=w334:i32)  [unwired: 11 in]
      n180 = call "myRIO_BRig_RT_dataMTrig_Solenoid_c__R.vi"() -> ("output_Solenoid_c__R"=w315:i32)  [unwired: 11 in]
      n181 = call "myRIO_BRig_RT_dataMTrig_Solenoid_Tcycle__R.vi"() -> ("output_Solenoid_Tcycle__R"=w318:i32)  [unwired: 11 in]
      n182 = call "myRIO_BRig_RT_dataMTrig_Audio_c__R.vi"() -> ("output_Audio_c__R"=w299:i32)  [unwired: 11 in]
      n183 = call "myRIO_BRig_RT_dataMTrig_Audio_Tcycle__R.vi"() -> ("output_Audio_Tcycle__R"=w298:i32)  [unwired: 11 in]
      n184 = Index Array(array=w328, index #1=w323, index #2=w334, index #3=w315, index #4=w318, index #5=w299, index #6=w298) -> (element #1=w333:u16, element #2=w332:u16, element #3=w317:u16, element #4=w316:u16, element #5=w297:u16, element #6=w296:u16)
      n185 = Add(x=w306, y=w333) -> (x+y=w330:u16)
      n186 = Add(x=w306, y=w317) -> (x+y=w321:u16)
      n187 = Add(x=w306, y=w297) -> (x+y=w309:u16)
      n188 = Less?(x=w330, y=w332) -> (x < y?=w303:bool)
      n189 = Less?(x=w321, y=w316) -> (x < y?=w304:bool)
      n190 = Less?(x=w309, y=w296) -> (x < y?=w305:bool)
      n191 = Decrement(x=w325) -> (x-1=w331:u16)
      n192 = Decrement(x=w319) -> (x-1=w322:u16)
      n193 = Decrement(x=w307) -> (x-1=w310:u16)
      n194 = Select(t=w330, s=w303, f=u16 0) -> (s? t:f=w326:u16)
      n195 = Select(t=w325, s=w303, f=w331) -> (s? t:f=w327:u16)
      n196 = Select(t=w321, s=w304, f=u16 0) -> (s? t:f=w314:u16)
      n197 = Select(t=w319, s=w304, f=w322) -> (s? t:f=w312:u16)
      n198 = Select(t=w309, s=w305, f=u16 0) -> (s? t:f=w302:u16)
      n199 = Select(t=w307, s=w305, f=w310) -> (s? t:f=w300:u16)
      n200 = Replace Array Subset(array=w328, new element #1=w326, index #1=w323, new element #2=w327, index #2=w324, new element #3=w314, index #3=w315, new element #4=w312, index #4=w313, new element #5=w302, index #5=w299, new element #6=w300, index #6=w301) -> (w311:u16[])
    }
    frame 12 {
      # "Audio_R"
      # "Tcycle"
      # "count"
      # "Audio_L"
      # "Tcycle"
      # "count"
      n201 = call "myRIO_BRig_RT_dataMTrig_Audio_c__L.vi"() -> ("output_Audio_c__L"=w349:i32)  [unwired: 11 in]
      n202 = call "myRIO_BRig_RT_dataMTrig_Audio_Tcycle__L.vi"() -> ("output_Audio_Tcycle__L"=w355:i32)  [unwired: 11 in]
      n203 = call "myRIO_BRig_RT_dataMTrig_Audio_c__R.vi"() -> ("output_Audio_c__R"=w341:i32)  [unwired: 11 in]
      n204 = call "myRIO_BRig_RT_dataMTrig_Audio_Tcycle__R.vi"() -> ("output_Audio_Tcycle__R"=w342:i32)  [unwired: 11 in]
      n205 = Index Array(array=w361, index #1=w349, index #2=w355, index #3=w341, index #4=w342) -> (element #1=w354:u16, element #2=w353:u16, element #3=w344:u16, element #4=w343:u16)
      n206 = Add(x=w337, y=w354) -> (x+y=w358:u16)
      n207 = Add(x=w337, y=w344) -> (x+y=w347:u16)
      n208 = Less?(x=w358, y=w353) -> (x < y?=w335:bool)
      n209 = Less?(x=w347, y=w343) -> (x < y?=w336:bool)
      n210 = Decrement(x=w356) -> (x-1=w359:u16)
      n211 = Decrement(x=w345) -> (x-1=w348:u16)
      n212 = Select(t=w358, s=w335, f=u16 0) -> (s? t:f=w352:u16)
      n213 = Select(t=w356, s=w335, f=w359) -> (s? t:f=w351:u16)
      n214 = Select(t=w347, s=w336, f=u16 0) -> (s? t:f=w339:u16)
      n215 = Select(t=w345, s=w336, f=w348) -> (s? t:f=w338:u16)
      n216 = Replace Array Subset(array=w361, new element #1=w352, index #1=w349, new element #2=w351, index #2=w350, new element #3=w339, index #3=w341, new element #4=w338, index #4=w340) -> (w360:u16[])
    }
    frame 13 {
      # "Audio_R"
      # "Tcycle"
      # "count"
      # "Audio_L"
      # "Tcycle"
      # "count"
      # "Solenoid__L"
      # "Tcycle"
      # "count"
      n217 = call "myRIO_BRig_RT_dataMTrig_Solenoid_c__L.vi"() -> ("output_Solenoid_c__L"=w365:i32)  [unwired: 11 in]
      n218 = call "myRIO_BRig_RT_dataMTrig_Solenoid_Tcycle__L.vi"() -> ("output_Solenoid_Tcycle__L"=w368:i32)  [unwired: 11 in]
      n219 = call "myRIO_BRig_RT_dataMTrig_Audio_c__L.vi"() -> ("output_Audio_c__L"=w384:i32)  [unwired: 11 in]
      n220 = call "myRIO_BRig_RT_dataMTrig_Audio_Tcycle__L.vi"() -> ("output_Audio_Tcycle__L"=w390:i32)  [unwired: 11 in]
      n221 = call "myRIO_BRig_RT_dataMTrig_Audio_c__R.vi"() -> ("output_Audio_c__R"=w376:i32)  [unwired: 11 in]
      n222 = call "myRIO_BRig_RT_dataMTrig_Audio_Tcycle__R.vi"() -> ("output_Audio_Tcycle__R"=w377:i32)  [unwired: 11 in]
      n223 = Index Array(array=w397, index #1=w365, index #2=w368, index #3=w384, index #4=w390, index #5=w376, index #6=w377) -> (element #1=w367:u16, element #2=w366:u16, element #3=w389:u16, element #4=w388:u16, element #5=w379:u16, element #6=w378:u16)
      n224 = Add(x=w372, y=w367) -> (x+y=w399:u16)
      n225 = Add(x=w372, y=w389) -> (x+y=w393:u16)
      n226 = Add(x=w372, y=w379) -> (x+y=w382:u16)
      n227 = Less?(x=w399, y=w366) -> (x < y?=w369:bool)
      n228 = Less?(x=w393, y=w388) -> (x < y?=w370:bool)
      n229 = Less?(x=w382, y=w378) -> (x < y?=w371:bool)
      n230 = Decrement(x=w396) -> (x-1=w400:u16)
      n231 = Decrement(x=w391) -> (x-1=w394:u16)
      n232 = Decrement(x=w380) -> (x-1=w383:u16)
      n233 = Select(t=w399, s=w369, f=u16 0) -> (s? t:f=w364:u16)
      n234 = Select(t=w396, s=w369, f=w400) -> (s? t:f=w362:u16)
      n235 = Select(t=w393, s=w370, f=u16 0) -> (s? t:f=w387:u16)
      n236 = Select(t=w391, s=w370, f=w394) -> (s? t:f=w386:u16)
      n237 = Select(t=w382, s=w371, f=u16 0) -> (s? t:f=w374:u16)
      n238 = Select(t=w380, s=w371, f=w383) -> (s? t:f=w373:u16)
      n239 = Replace Array Subset(array=w397, new element #1=w364, index #1=w365, new element #2=w362, index #2=w363, new element #3=w387, index #3=w384, new element #4=w386, index #4=w385, new element #5=w374, index #5=w376, new element #6=w373, index #6=w375) -> (w395:u16[])
    }
    frame 14 {
      # "Audio_R"
      # "Tcycle"
      # "count"
      # "Audio_L"
      # "Tcycle"
      # "count"
      # "Solenoid__R"
      # "Tcycle"
      # "count"
      n240 = call "myRIO_BRig_RT_dataMTrig_Solenoid_c__R.vi"() -> ("output_Solenoid_c__R"=w431:i32)  [unwired: 11 in]
      n241 = call "myRIO_BRig_RT_dataMTrig_Solenoid_Tcycle__R.vi"() -> ("output_Solenoid_Tcycle__R"=w434:i32)  [unwired: 11 in]
      n242 = call "myRIO_BRig_RT_dataMTrig_Audio_c__L.vi"() -> ("output_Audio_c__L"=w416:i32)  [unwired: 11 in]
      n243 = call "myRIO_BRig_RT_dataMTrig_Audio_Tcycle__L.vi"() -> ("output_Audio_Tcycle__L"=w422:i32)  [unwired: 11 in]
      n244 = call "myRIO_BRig_RT_dataMTrig_Audio_c__R.vi"() -> ("output_Audio_c__R"=w408:i32)  [unwired: 11 in]
      n245 = call "myRIO_BRig_RT_dataMTrig_Audio_Tcycle__R.vi"() -> ("output_Audio_Tcycle__R"=w409:i32)  [unwired: 11 in]
      n246 = Index Array(array=w439, index #1=w431, index #2=w434, index #3=w416, index #4=w422, index #5=w408, index #6=w409) -> (element #1=w433:u16, element #2=w432:u16, element #3=w421:u16, element #4=w420:u16, element #5=w411:u16, element #6=w410:u16)
      n247 = Add(x=w404, y=w433) -> (x+y=w437:u16)
      n248 = Add(x=w404, y=w421) -> (x+y=w425:u16)
      n249 = Add(x=w404, y=w411) -> (x+y=w414:u16)
      n250 = Less?(x=w437, y=w432) -> (x < y?=w401:bool)
      n251 = Less?(x=w425, y=w420) -> (x < y?=w402:bool)
      n252 = Less?(x=w414, y=w410) -> (x < y?=w403:bool)
      n253 = Decrement(x=w435) -> (x-1=w438:u16)
      n254 = Decrement(x=w423) -> (x-1=w426:u16)
      n255 = Decrement(x=w412) -> (x-1=w415:u16)
      n256 = Select(t=w437, s=w401, f=u16 0) -> (s? t:f=w430:u16)
      n257 = Select(t=w435, s=w401, f=w438) -> (s? t:f=w428:u16)
      n258 = Select(t=w425, s=w402, f=u16 0) -> (s? t:f=w419:u16)
      n259 = Select(t=w423, s=w402, f=w426) -> (s? t:f=w418:u16)
      n260 = Select(t=w414, s=w403, f=u16 0) -> (s? t:f=w406:u16)
      n261 = Select(t=w412, s=w403, f=w415) -> (s? t:f=w405:u16)
      n262 = Replace Array Subset(array=w439, new element #1=w430, index #1=w431, new element #2=w428, index #2=w429, new element #3=w419, index #3=w416, new element #4=w418, index #4=w417, new element #5=w406, index #5=w408, new element #6=w405, index #6=w407) -> (w427:u16[])
    }
    frame 15 {
      # "Audio_R"
      # "Tcycle"
      # "count"
      # "Audio_L"
      # "Tcycle"
      # "count"
      # "Solenoid__R"
      # "Tcycle"
      # "count"
      # "Solenoid__L"
      # "Tcycle"
      # "count"
      n263 = call "myRIO_BRig_RT_dataMTrig_Solenoid_c__L.vi"() -> ("output_Solenoid_c__L"=w479:i32)  [unwired: 11 in]
      n264 = call "myRIO_BRig_RT_dataMTrig_Solenoid_Tcycle__L.vi"() -> ("output_Solenoid_Tcycle__L"=w490:i32)  [unwired: 11 in]
      n265 = call "myRIO_BRig_RT_dataMTrig_Solenoid_c__R.vi"() -> ("output_Solenoid_c__R"=w471:i32)  [unwired: 11 in]
      n266 = call "myRIO_BRig_RT_dataMTrig_Solenoid_Tcycle__R.vi"() -> ("output_Solenoid_Tcycle__R"=w474:i32)  [unwired: 11 in]
      n267 = call "myRIO_BRig_RT_dataMTrig_Audio_c__L.vi"() -> ("output_Audio_c__L"=w456:i32)  [unwired: 11 in]
      n268 = call "myRIO_BRig_RT_dataMTrig_Audio_Tcycle__L.vi"() -> ("output_Audio_Tcycle__L"=w462:i32)  [unwired: 11 in]
      n269 = call "myRIO_BRig_RT_dataMTrig_Audio_c__R.vi"() -> ("output_Audio_c__R"=w448:i32)  [unwired: 11 in]
      n270 = call "myRIO_BRig_RT_dataMTrig_Audio_Tcycle__R.vi"() -> ("output_Audio_Tcycle__R"=w449:i32)  [unwired: 11 in]
      n271 = Index Array(array=w484, index #1=w479, index #2=w490, index #3=w471, index #4=w474, index #5=w456, index #6=w462, index #7=w448, index #8=w449) -> (element #1=w489:u16, element #2=w488:u16, element #3=w473:u16, element #4=w472:u16, element #5=w461:u16, element #6=w460:u16, element #7=w451:u16, element #8=w450:u16)
      n272 = Add(x=w444, y=w489) -> (x+y=w486:u16)
      n273 = Add(x=w444, y=w473) -> (x+y=w477:u16)
      n274 = Add(x=w444, y=w461) -> (x+y=w465:u16)
      n275 = Add(x=w444, y=w451) -> (x+y=w454:u16)
      n276 = Less?(x=w486, y=w488) -> (x < y?=w440:bool)
      n277 = Less?(x=w477, y=w472) -> (x < y?=w441:bool)
      n278 = Less?(x=w465, y=w460) -> (x < y?=w442:bool)
      n279 = Less?(x=w454, y=w450) -> (x < y?=w443:bool)
      n280 = Decrement(x=w481) -> (x-1=w487:u16)
      n281 = Decrement(x=w475) -> (x-1=w478:u16)
      n282 = Decrement(x=w463) -> (x-1=w466:u16)
      n283 = Decrement(x=w452) -> (x-1=w455:u16)
      n284 = Select(t=w486, s=w440, f=u16 0) -> (s? t:f=w482:u16)
      n285 = Select(t=w481, s=w440, f=w487) -> (s? t:f=w483:u16)
      n286 = Select(t=w477, s=w441, f=u16 0) -> (s? t:f=w470:u16)
      n287 = Select(t=w475, s=w441, f=w478) -> (s? t:f=w468:u16)
      n288 = Select(t=w465, s=w442, f=u16 0) -> (s? t:f=w459:u16)
      n289 = Select(t=w463, s=w442, f=w466) -> (s? t:f=w458:u16)
      n290 = Select(t=w454, s=w443, f=u16 0) -> (s? t:f=w446:u16)
      n291 = Select(t=w452, s=w443, f=w455) -> (s? t:f=w445:u16)
      n292 = Replace Array Subset(array=w484, new element #1=w482, index #1=w479, new element #2=w483, index #2=w480, new element #3=w470, index #3=w471, new element #4=w468, index #4=w469, new element #5=w459, index #5=w456, new element #6=w458, index #6=w457, new element #7=w446, index #7=w448, new element #8=w445, index #8=w447) -> (w467:u16[])
    }
    frame 16 {
      # "Laser"
      # "Tcycle"
      # "count"
      n293 = call "myRIO_BRig_RT_dataMTrig_Laser_c.vi"() -> ("output_Laser_c"=w495:i32)  [unwired: 11 in]
      n294 = call "myRIO_BRig_RT_dataMTrig_Laser_Tcycle.vi"() -> ("output_Laser_Tcycle"=w498:i32)  [unwired: 11 in]
      n295 = Index Array(array=w505, index #1=w495, index #2=w498) -> (element #1=w497:u16, element #2=w496:u16)
      n296 = Add(x=w499, y=w497) -> (x+y=w502:u16)
      n297 = Less?(x=w502, y=w496) -> (x < y?=w491:bool)
      n298 = Decrement(x=w500) -> (x-1=w503:u16)
      n299 = Select(t=w502, s=w491, f=u16 0) -> (s? t:f=w493:u16)
      n300 = Select(t=w500, s=w491, f=w503) -> (s? t:f=w492:u16)
      n301 = Replace Array Subset(array=w505, new element #1=w493, index #1=w495, new element #2=w492, index #2=w494) -> (w504:u16[])
    }
    frame 17 {
      # "Laser"
      # "Tcycle"
      # "count"
      # "Solenoid__L"
      # "Tcycle"
      # "count"
      n302 = call "myRIO_BRig_RT_dataMTrig_Solenoid_c__L.vi"() -> ("output_Solenoid_c__L"=w521:i32)  [unwired: 11 in]
      n303 = call "myRIO_BRig_RT_dataMTrig_Solenoid_Tcycle__L.vi"() -> ("output_Solenoid_Tcycle__L"=w532:i32)  [unwired: 11 in]
      n304 = call "myRIO_BRig_RT_dataMTrig_Laser_c.vi"() -> ("output_Laser_c"=w509:i32)  [unwired: 11 in]
      n305 = call "myRIO_BRig_RT_dataMTrig_Laser_Tcycle.vi"() -> ("output_Laser_Tcycle"=w512:i32)  [unwired: 11 in]
      n306 = Index Array(array=w526, index #1=w521, index #2=w532, index #3=w509, index #4=w512) -> (element #1=w531:u16, element #2=w530:u16, element #3=w511:u16, element #4=w510:u16)
      n307 = Add(x=w515, y=w531) -> (x+y=w528:u16)
      n308 = Add(x=w515, y=w511) -> (x+y=w518:u16)
      n309 = Less?(x=w528, y=w530) -> (x < y?=w513:bool)
      n310 = Less?(x=w518, y=w510) -> (x < y?=w514:bool)
      n311 = Decrement(x=w523) -> (x-1=w529:u16)
      n312 = Decrement(x=w516) -> (x-1=w519:u16)
      n313 = Select(t=w528, s=w513, f=u16 0) -> (s? t:f=w524:u16)
      n314 = Select(t=w523, s=w513, f=w529) -> (s? t:f=w525:u16)
      n315 = Select(t=w518, s=w514, f=u16 0) -> (s? t:f=w508:u16)
      n316 = Select(t=w516, s=w514, f=w519) -> (s? t:f=w506:u16)
      n317 = Replace Array Subset(array=w526, new element #1=w524, index #1=w521, new element #2=w525, index #2=w522, new element #3=w508, index #3=w509, new element #4=w506, index #4=w507) -> (w520:u16[])
    }
    frame 18 {
      # "Laser"
      # "Tcycle"
      # "count"
      # "Solenoid__R"
      # "Tcycle"
      # "count"
      n318 = call "myRIO_BRig_RT_dataMTrig_Solenoid_c__R.vi"() -> ("output_Solenoid_c__R"=w551:i32)  [unwired: 11 in]
      n319 = call "myRIO_BRig_RT_dataMTrig_Solenoid_Tcycle__R.vi"() -> ("output_Solenoid_Tcycle__R"=w554:i32)  [unwired: 11 in]
      n320 = call "myRIO_BRig_RT_dataMTrig_Laser_c.vi"() -> ("output_Laser_c"=w536:i32)  [unwired: 11 in]
      n321 = call "myRIO_BRig_RT_dataMTrig_Laser_Tcycle.vi"() -> ("output_Laser_Tcycle"=w539:i32)  [unwired: 11 in]
      n322 = Index Array(array=w559, index #1=w551, index #2=w554, index #3=w536, index #4=w539) -> (element #1=w553:u16, element #2=w552:u16, element #3=w538:u16, element #4=w537:u16)
      n323 = Add(x=w542, y=w553) -> (x+y=w557:u16)
      n324 = Add(x=w542, y=w538) -> (x+y=w545:u16)
      n325 = Less?(x=w557, y=w552) -> (x < y?=w540:bool)
      n326 = Less?(x=w545, y=w537) -> (x < y?=w541:bool)
      n327 = Decrement(x=w555) -> (x-1=w558:u16)
      n328 = Decrement(x=w543) -> (x-1=w546:u16)
      n329 = Select(t=w557, s=w540, f=u16 0) -> (s? t:f=w550:u16)
      n330 = Select(t=w555, s=w540, f=w558) -> (s? t:f=w548:u16)
      n331 = Select(t=w545, s=w541, f=u16 0) -> (s? t:f=w535:u16)
      n332 = Select(t=w543, s=w541, f=w546) -> (s? t:f=w533:u16)
      n333 = Replace Array Subset(array=w559, new element #1=w550, index #1=w551, new element #2=w548, index #2=w549, new element #3=w535, index #3=w536, new element #4=w533, index #4=w534) -> (w547:u16[])
    }
    frame 19 {
      # "Laser"
      # "Tcycle"
      # "count"
      # "Solenoid__R"
      # "Tcycle"
      # "count"
      # "Solenoid__L"
      # "Tcycle"
      # "count"
      n334 = call "myRIO_BRig_RT_dataMTrig_Solenoid_c__L.vi"() -> ("output_Solenoid_c__L"=w587:i32)  [unwired: 11 in]
      n335 = call "myRIO_BRig_RT_dataMTrig_Solenoid_Tcycle__L.vi"() -> ("output_Solenoid_Tcycle__L"=w598:i32)  [unwired: 11 in]
      n336 = call "myRIO_BRig_RT_dataMTrig_Solenoid_c__R.vi"() -> ("output_Solenoid_c__R"=w579:i32)  [unwired: 11 in]
      n337 = call "myRIO_BRig_RT_dataMTrig_Solenoid_Tcycle__R.vi"() -> ("output_Solenoid_Tcycle__R"=w582:i32)  [unwired: 11 in]
      n338 = call "myRIO_BRig_RT_dataMTrig_Laser_c.vi"() -> ("output_Laser_c"=w563:i32)  [unwired: 11 in]
      n339 = call "myRIO_BRig_RT_dataMTrig_Laser_Tcycle.vi"() -> ("output_Laser_Tcycle"=w566:i32)  [unwired: 11 in]
      n340 = Index Array(array=w592, index #1=w587, index #2=w598, index #3=w579, index #4=w582, index #5=w563, index #6=w566) -> (element #1=w597:u16, element #2=w596:u16, element #3=w581:u16, element #4=w580:u16, element #5=w565:u16, element #6=w564:u16)
      n341 = Add(x=w570, y=w597) -> (x+y=w594:u16)
      n342 = Add(x=w570, y=w581) -> (x+y=w585:u16)
      n343 = Add(x=w570, y=w565) -> (x+y=w573:u16)
      n344 = Less?(x=w594, y=w596) -> (x < y?=w567:bool)
      n345 = Less?(x=w585, y=w580) -> (x < y?=w568:bool)
      n346 = Less?(x=w573, y=w564) -> (x < y?=w569:bool)
      n347 = Decrement(x=w589) -> (x-1=w595:u16)
      n348 = Decrement(x=w583) -> (x-1=w586:u16)
      n349 = Decrement(x=w571) -> (x-1=w574:u16)
      n350 = Select(t=w594, s=w567, f=u16 0) -> (s? t:f=w590:u16)
      n351 = Select(t=w589, s=w567, f=w595) -> (s? t:f=w591:u16)
      n352 = Select(t=w585, s=w568, f=u16 0) -> (s? t:f=w578:u16)
      n353 = Select(t=w583, s=w568, f=w586) -> (s? t:f=w576:u16)
      n354 = Select(t=w573, s=w569, f=u16 0) -> (s? t:f=w562:u16)
      n355 = Select(t=w571, s=w569, f=w574) -> (s? t:f=w560:u16)
      n356 = Replace Array Subset(array=w592, new element #1=w590, index #1=w587, new element #2=w591, index #2=w588, new element #3=w578, index #3=w579, new element #4=w576, index #4=w577, new element #5=w562, index #5=w563, new element #6=w560, index #6=w561) -> (w575:u16[])
    }
    frame 20 {
      # "Laser"
      # "Tcycle"
      # "count"
      # "Audio_L"
      # "Tcycle"
      # "count"
      n357 = call "myRIO_BRig_RT_dataMTrig_Audio_c__L.vi"() -> ("output_Audio_c__L"=w613:i32)  [unwired: 11 in]
      n358 = call "myRIO_BRig_RT_dataMTrig_Audio_Tcycle__L.vi"() -> ("output_Audio_Tcycle__L"=w619:i32)  [unwired: 11 in]
      n359 = call "myRIO_BRig_RT_dataMTrig_Laser_c.vi"() -> ("output_Laser_c"=w602:i32)  [unwired: 11 in]
      n360 = call "myRIO_BRig_RT_dataMTrig_Laser_Tcycle.vi"() -> ("output_Laser_Tcycle"=w605:i32)  [unwired: 11 in]
      n361 = Index Array(array=w625, index #1=w613, index #2=w619, index #3=w602, index #4=w605) -> (element #1=w618:u16, element #2=w617:u16, element #3=w604:u16, element #4=w603:u16)
      n362 = Add(x=w608, y=w618) -> (x+y=w622:u16)
      n363 = Add(x=w608, y=w604) -> (x+y=w611:u16)
      n364 = Less?(x=w622, y=w617) -> (x < y?=w606:bool)
      n365 = Less?(x=w611, y=w603) -> (x < y?=w607:bool)
      n366 = Decrement(x=w620) -> (x-1=w623:u16)
      n367 = Decrement(x=w609) -> (x-1=w612:u16)
      n368 = Select(t=w622, s=w606, f=u16 0) -> (s? t:f=w616:u16)
      n369 = Select(t=w620, s=w606, f=w623) -> (s? t:f=w615:u16)
      n370 = Select(t=w611, s=w607, f=u16 0) -> (s? t:f=w601:u16)
      n371 = Select(t=w609, s=w607, f=w612) -> (s? t:f=w599:u16)
      n372 = Replace Array Subset(array=w625, new element #1=w616, index #1=w613, new element #2=w615, index #2=w614, new element #3=w601, index #3=w602, new element #4=w599, index #4=w600) -> (w624:u16[])
    }
    frame 21 {
      # "Laser"
      # "Tcycle"
      # "count"
      # "Audio_L"
      # "Tcycle"
      # "count"
      # "Solenoid__L"
      # "Tcycle"
      # "count"
      n373 = call "myRIO_BRig_RT_dataMTrig_Solenoid_c__L.vi"() -> ("output_Solenoid_c__L"=w653:i32)  [unwired: 11 in]
      n374 = call "myRIO_BRig_RT_dataMTrig_Solenoid_Tcycle__L.vi"() -> ("output_Solenoid_Tcycle__L"=w664:i32)  [unwired: 11 in]
      n375 = call "myRIO_BRig_RT_dataMTrig_Audio_c__L.vi"() -> ("output_Audio_c__L"=w633:i32)  [unwired: 11 in]
      n376 = call "myRIO_BRig_RT_dataMTrig_Audio_Tcycle__L.vi"() -> ("output_Audio_Tcycle__L"=w639:i32)  [unwired: 11 in]
      n377 = call "myRIO_BRig_RT_dataMTrig_Laser_c.vi"() -> ("output_Laser_c"=w629:i32)  [unwired: 11 in]
      n378 = call "myRIO_BRig_RT_dataMTrig_Laser_Tcycle.vi"() -> ("output_Laser_Tcycle"=w638:i32)  [unwired: 11 in]
      n379 = Index Array(array=w658, index #1=w653, index #2=w664, index #3=w633, index #4=w639, index #5=w629, index #6=w638) -> (element #1=w663:u16, element #2=w662:u16, element #3=w637:u16, element #4=w636:u16, element #5=w635:u16, element #6=w634:u16)
      n380 = Add(x=w643, y=w663) -> (x+y=w660:u16)
      n381 = Add(x=w643, y=w637) -> (x+y=w650:u16)
      n382 = Add(x=w643, y=w635) -> (x+y=w646:u16)
      n383 = Less?(x=w660, y=w662) -> (x < y?=w640:bool)
      n384 = Less?(x=w650, y=w636) -> (x < y?=w641:bool)
      n385 = Less?(x=w646, y=w634) -> (x < y?=w642:bool)
      n386 = Decrement(x=w655) -> (x-1=w661:u16)
      n387 = Decrement(x=w648) -> (x-1=w651:u16)
      n388 = Decrement(x=w644) -> (x-1=w647:u16)
      n389 = Select(t=w660, s=w640, f=u16 0) -> (s? t:f=w656:u16)
      n390 = Select(t=w655, s=w640, f=w661) -> (s? t:f=w657:u16)
      n391 = Select(t=w650, s=w641, f=u16 0) -> (s? t:f=w632:u16)
      n392 = Select(t=w648, s=w641, f=w651) -> (s? t:f=w630:u16)
      n393 = Select(t=w646, s=w642, f=u16 0) -> (s? t:f=w628:u16)
      n394 = Select(t=w644, s=w642, f=w647) -> (s? t:f=w626:u16)
      n395 = Replace Array Subset(array=w658, new element #1=w656, index #1=w653, new element #2=w657, index #2=w654, new element #3=w632, index #3=w633, new element #4=w630, index #4=w631, new element #5=w628, index #5=w629, new element #6=w626, index #6=w627) -> (w652:u16[])
    }
    frame 22 {
      # "Laser"
      # "Tcycle"
      # "count"
      # "Audio_L"
      # "Tcycle"
      # "count"
      # "Solenoid__R"
      # "Tcycle"
      # "count"
      n396 = call "myRIO_BRig_RT_dataMTrig_Solenoid_c__R.vi"() -> ("output_Solenoid_c__R"=w695:i32)  [unwired: 11 in]
      n397 = call "myRIO_BRig_RT_dataMTrig_Solenoid_Tcycle__R.vi"() -> ("output_Solenoid_Tcycle__R"=w698:i32)  [unwired: 11 in]
      n398 = call "myRIO_BRig_RT_dataMTrig_Audio_c__L.vi"() -> ("output_Audio_c__L"=w680:i32)  [unwired: 11 in]
      n399 = call "myRIO_BRig_RT_dataMTrig_Audio_Tcycle__L.vi"() -> ("output_Audio_Tcycle__L"=w686:i32)  [unwired: 11 in]
      n400 = call "myRIO_BRig_RT_dataMTrig_Laser_c.vi"() -> ("output_Laser_c"=w668:i32)  [unwired: 11 in]
      n401 = call "myRIO_BRig_RT_dataMTrig_Laser_Tcycle.vi"() -> ("output_Laser_Tcycle"=w671:i32)  [unwired: 11 in]
      n402 = Index Array(array=w703, index #1=w695, index #2=w698, index #3=w680, index #4=w686, index #5=w668, index #6=w671) -> (element #1=w697:u16, element #2=w696:u16, element #3=w685:u16, element #4=w684:u16, element #5=w670:u16, element #6=w669:u16)
      n403 = Add(x=w675, y=w697) -> (x+y=w701:u16)
      n404 = Add(x=w675, y=w685) -> (x+y=w689:u16)
      n405 = Add(x=w675, y=w670) -> (x+y=w678:u16)
      n406 = Less?(x=w701, y=w696) -> (x < y?=w672:bool)
      n407 = Less?(x=w689, y=w684) -> (x < y?=w673:bool)
      n408 = Less?(x=w678, y=w669) -> (x < y?=w674:bool)
      n409 = Decrement(x=w699) -> (x-1=w702:u16)
      n410 = Decrement(x=w687) -> (x-1=w690:u16)
      n411 = Decrement(x=w676) -> (x-1=w679:u16)
      n412 = Select(t=w701, s=w672, f=u16 0) -> (s? t:f=w694:u16)
      n413 = Select(t=w699, s=w672, f=w702) -> (s? t:f=w692:u16)
      n414 = Select(t=w689, s=w673, f=u16 0) -> (s? t:f=w683:u16)
      n415 = Select(t=w687, s=w673, f=w690) -> (s? t:f=w682:u16)
      n416 = Select(t=w678, s=w674, f=u16 0) -> (s? t:f=w667:u16)
      n417 = Select(t=w676, s=w674, f=w679) -> (s? t:f=w665:u16)
      n418 = Replace Array Subset(array=w703, new element #1=w694, index #1=w695, new element #2=w692, index #2=w693, new element #3=w683, index #3=w680, new element #4=w682, index #4=w681, new element #5=w667, index #5=w668, new element #6=w665, index #6=w666) -> (w691:u16[])
    }
    frame 23 {
      # "Laser"
      # "Tcycle"
      # "count"
      # "Audio_L"
      # "Tcycle"
      # "count"
      # "Solenoid__R"
      # "Tcycle"
      # "count"
      # "Solenoid__L"
      # "Tcycle"
      # "count"
      n419 = call "myRIO_BRig_RT_dataMTrig_Solenoid_c__L.vi"() -> ("output_Solenoid_c__L"=w743:i32)  [unwired: 11 in]
      n420 = call "myRIO_BRig_RT_dataMTrig_Solenoid_Tcycle__L.vi"() -> ("output_Solenoid_Tcycle__L"=w754:i32)  [unwired: 11 in]
      n421 = call "myRIO_BRig_RT_dataMTrig_Solenoid_c__R.vi"() -> ("output_Solenoid_c__R"=w735:i32)  [unwired: 11 in]
      n422 = call "myRIO_BRig_RT_dataMTrig_Solenoid_Tcycle__R.vi"() -> ("output_Solenoid_Tcycle__R"=w738:i32)  [unwired: 11 in]
      n423 = call "myRIO_BRig_RT_dataMTrig_Audio_c__L.vi"() -> ("output_Audio_c__L"=w720:i32)  [unwired: 11 in]
      n424 = call "myRIO_BRig_RT_dataMTrig_Audio_Tcycle__L.vi"() -> ("output_Audio_Tcycle__L"=w726:i32)  [unwired: 11 in]
      n425 = call "myRIO_BRig_RT_dataMTrig_Laser_c.vi"() -> ("output_Laser_c"=w707:i32)  [unwired: 11 in]
      n426 = call "myRIO_BRig_RT_dataMTrig_Laser_Tcycle.vi"() -> ("output_Laser_Tcycle"=w710:i32)  [unwired: 11 in]
      n427 = Index Array(array=w748, index #1=w743, index #2=w754, index #3=w735, index #4=w738, index #5=w720, index #6=w726, index #7=w707, index #8=w710) -> (element #1=w753:u16, element #2=w752:u16, element #3=w737:u16, element #4=w736:u16, element #5=w725:u16, element #6=w724:u16, element #7=w709:u16, element #8=w708:u16)
      n428 = Add(x=w715, y=w753) -> (x+y=w750:u16)
      n429 = Add(x=w715, y=w737) -> (x+y=w741:u16)
      n430 = Add(x=w715, y=w725) -> (x+y=w729:u16)
      n431 = Add(x=w715, y=w709) -> (x+y=w718:u16)
      n432 = Less?(x=w750, y=w752) -> (x < y?=w711:bool)
      n433 = Less?(x=w741, y=w736) -> (x < y?=w712:bool)
      n434 = Less?(x=w729, y=w724) -> (x < y?=w713:bool)
      n435 = Less?(x=w718, y=w708) -> (x < y?=w714:bool)
      n436 = Decrement(x=w745) -> (x-1=w751:u16)
      n437 = Decrement(x=w739) -> (x-1=w742:u16)
      n438 = Decrement(x=w727) -> (x-1=w730:u16)
      n439 = Decrement(x=w716) -> (x-1=w719:u16)
      n440 = Select(t=w750, s=w711, f=u16 0) -> (s? t:f=w746:u16)
      n441 = Select(t=w745, s=w711, f=w751) -> (s? t:f=w747:u16)
      n442 = Select(t=w741, s=w712, f=u16 0) -> (s? t:f=w734:u16)
      n443 = Select(t=w739, s=w712, f=w742) -> (s? t:f=w732:u16)
      n444 = Select(t=w729, s=w713, f=u16 0) -> (s? t:f=w723:u16)
      n445 = Select(t=w727, s=w713, f=w730) -> (s? t:f=w722:u16)
      n446 = Select(t=w718, s=w714, f=u16 0) -> (s? t:f=w706:u16)
      n447 = Select(t=w716, s=w714, f=w719) -> (s? t:f=w704:u16)
      n448 = Replace Array Subset(array=w748, new element #1=w746, index #1=w743, new element #2=w747, index #2=w744, new element #3=w734, index #3=w735, new element #4=w732, index #4=w733, new element #5=w723, index #5=w720, new element #6=w722, index #6=w721, new element #7=w706, index #7=w707, new element #8=w704, index #8=w705) -> (w731:u16[])
    }
    frame 24 {
      # "Laser"
      # "Tcycle"
      # "count"
      # "Audio_R"
      # "Tcycle"
      # "count"
      n449 = call "myRIO_BRig_RT_dataMTrig_Audio_c__R.vi"() -> ("output_Audio_c__R"=w772:i32)  [unwired: 11 in]
      n450 = call "myRIO_BRig_RT_dataMTrig_Audio_Tcycle__R.vi"() -> ("output_Audio_Tcycle__R"=w773:i32)  [unwired: 11 in]
      n451 = call "myRIO_BRig_RT_dataMTrig_Laser_c.vi"() -> ("output_Laser_c"=w760:i32)  [unwired: 11 in]
      n452 = call "myRIO_BRig_RT_dataMTrig_Laser_Tcycle.vi"() -> ("output_Laser_Tcycle"=w763:i32)  [unwired: 11 in]
      n453 = Index Array(array=w781, index #1=w772, index #2=w773, index #3=w760, index #4=w763) -> (element #1=w775:u16, element #2=w774:u16, element #3=w762:u16, element #4=w761:u16)
      n454 = Add(x=w764, y=w775) -> (x+y=w778:u16)
      n455 = Add(x=w764, y=w762) -> (x+y=w767:u16)
      n456 = Less?(x=w778, y=w774) -> (x < y?=w755:bool)
      n457 = Less?(x=w767, y=w761) -> (x < y?=w756:bool)
      n458 = Decrement(x=w776) -> (x-1=w779:u16)
      n459 = Decrement(x=w765) -> (x-1=w768:u16)
      n460 = Select(t=w778, s=w755, f=u16 0) -> (s? t:f=w770:u16)
      n461 = Select(t=w776, s=w755, f=w779) -> (s? t:f=w769:u16)
      n462 = Select(t=w767, s=w756, f=u16 0) -> (s? t:f=w758:u16)
      n463 = Select(t=w765, s=w756, f=w768) -> (s? t:f=w757:u16)
      n464 = Replace Array Subset(array=w781, new element #1=w770, index #1=w772, new element #2=w769, index #2=w771, new element #3=w758, index #3=w760, new element #4=w757, index #4=w759) -> (w780:u16[])
    }
    frame 25 {
      # "Laser"
      # "Tcycle"
      # "count"
      # "Audio_R"
      # "Tcycle"
      # "count"
      # "Solenoid__L"
      # "Tcycle"
      # "count"
      n465 = call "myRIO_BRig_RT_dataMTrig_Solenoid_c__L.vi"() -> ("output_Solenoid_c__L"=w785:i32)  [unwired: 11 in]
      n466 = call "myRIO_BRig_RT_dataMTrig_Solenoid_Tcycle__L.vi"() -> ("output_Solenoid_Tcycle__L"=w788:i32)  [unwired: 11 in]
      n467 = call "myRIO_BRig_RT_dataMTrig_Audio_c__R.vi"() -> ("output_Audio_c__R"=w807:i32)  [unwired: 11 in]
      n468 = call "myRIO_BRig_RT_dataMTrig_Audio_Tcycle__R.vi"() -> ("output_Audio_Tcycle__R"=w808:i32)  [unwired: 11 in]
      n469 = call "myRIO_BRig_RT_dataMTrig_Laser_c.vi"() -> ("output_Laser_c"=w795:i32)  [unwired: 11 in]
      n470 = call "myRIO_BRig_RT_dataMTrig_Laser_Tcycle.vi"() -> ("output_Laser_Tcycle"=w798:i32)  [unwired: 11 in]
      n471 = Index Array(array=w817, index #1=w785, index #2=w788, index #3=w807, index #4=w808, index #5=w795, index #6=w798) -> (element #1=w787:u16, element #2=w786:u16, element #3=w810:u16, element #4=w809:u16, element #5=w797:u16, element #6=w796:u16)
      n472 = Add(x=w799, y=w787) -> (x+y=w819:u16)
      n473 = Add(x=w799, y=w810) -> (x+y=w813:u16)
      n474 = Add(x=w799, y=w797) -> (x+y=w802:u16)
      n475 = Less?(x=w819, y=w786) -> (x < y?=w789:bool)
      n476 = Less?(x=w813, y=w809) -> (x < y?=w790:bool)
      n477 = Less?(x=w802, y=w796) -> (x < y?=w791:bool)
      n478 = Decrement(x=w816) -> (x-1=w820:u16)
      n479 = Decrement(x=w811) -> (x-1=w814:u16)
      n480 = Decrement(x=w800) -> (x-1=w803:u16)
      n481 = Select(t=w819, s=w789, f=u16 0) -> (s? t:f=w784:u16)
      n482 = Select(t=w816, s=w789, f=w820) -> (s? t:f=w782:u16)
      n483 = Select(t=w813, s=w790, f=u16 0) -> (s? t:f=w805:u16)
      n484 = Select(t=w811, s=w790, f=w814) -> (s? t:f=w804:u16)
      n485 = Select(t=w802, s=w791, f=u16 0) -> (s? t:f=w793:u16)
      n486 = Select(t=w800, s=w791, f=w803) -> (s? t:f=w792:u16)
      n487 = Replace Array Subset(array=w817, new element #1=w784, index #1=w785, new element #2=w782, index #2=w783, new element #3=w805, index #3=w807, new element #4=w804, index #4=w806, new element #5=w793, index #5=w795, new element #6=w792, index #6=w794) -> (w815:u16[])
    }
    frame 26 {
      # "Laser"
      # "Tcycle"
      # "count"
      # "Audio_R"
      # "Tcycle"
      # "count"
      # "Solenoid__R"
      # "Tcycle"
      # "count"
      n488 = call "myRIO_BRig_RT_dataMTrig_Solenoid_c__R.vi"() -> ("output_Solenoid_c__R"=w822:i32)  [unwired: 11 in]
      n489 = call "myRIO_BRig_RT_dataMTrig_Solenoid_Tcycle__R.vi"() -> ("output_Solenoid_Tcycle__R"=w821:i32)  [unwired: 11 in]
      n490 = call "myRIO_BRig_RT_dataMTrig_Audio_c__R.vi"() -> ("output_Audio_c__R"=w846:i32)  [unwired: 11 in]
      n491 = call "myRIO_BRig_RT_dataMTrig_Audio_Tcycle__R.vi"() -> ("output_Audio_Tcycle__R"=w847:i32)  [unwired: 11 in]
      n492 = call "myRIO_BRig_RT_dataMTrig_Laser_c.vi"() -> ("output_Laser_c"=w834:i32)  [unwired: 11 in]
      n493 = call "myRIO_BRig_RT_dataMTrig_Laser_Tcycle.vi"() -> ("output_Laser_Tcycle"=w837:i32)  [unwired: 11 in]
      n494 = Index Array(array=w859, index #1=w822, index #2=w821, index #3=w846, index #4=w847, index #5=w834, index #6=w837) -> (element #1=w824:u16, element #2=w823:u16, element #3=w849:u16, element #4=w848:u16, element #5=w836:u16, element #6=w835:u16)
      n495 = Add(x=w838, y=w824) -> (x+y=w857:u16)
      n496 = Add(x=w838, y=w849) -> (x+y=w852:u16)
      n497 = Add(x=w838, y=w836) -> (x+y=w841:u16)
      n498 = Less?(x=w857, y=w823) -> (x < y?=w828:bool)
      n499 = Less?(x=w852, y=w848) -> (x < y?=w829:bool)
      n500 = Less?(x=w841, y=w835) -> (x < y?=w830:bool)
      n501 = Decrement(x=w855) -> (x-1=w858:u16)
      n502 = Decrement(x=w850) -> (x-1=w853:u16)
      n503 = Decrement(x=w839) -> (x-1=w842:u16)
      n504 = Select(t=w857, s=w828, f=u16 0) -> (s? t:f=w827:u16)
      n505 = Select(t=w855, s=w828, f=w858) -> (s? t:f=w825:u16)
      n506 = Select(t=w852, s=w829, f=u16 0) -> (s? t:f=w844:u16)
      n507 = Select(t=w850, s=w829, f=w853) -> (s? t:f=w843:u16)
      n508 = Select(t=w841, s=w830, f=u16 0) -> (s? t:f=w832:u16)
      n509 = Select(t=w839, s=w830, f=w842) -> (s? t:f=w831:u16)
      n510 = Replace Array Subset(array=w859, new element #1=w827, index #1=w822, new element #2=w825, index #2=w826, new element #3=w844, index #3=w846, new element #4=w843, index #4=w845, new element #5=w832, index #5=w834, new element #6=w831, index #6=w833) -> (w854:u16[])
    }
    frame 27 {
      # "Laser"
      # "Tcycle"
      # "count"
      # "Audio_R"
      # "Tcycle"
      # "count"
      # "Solenoid__R"
      # "Tcycle"
      # "count"
      # "Solenoid__L"
      # "Tcycle"
      # "count"
      n511 = call "myRIO_BRig_RT_dataMTrig_Solenoid_c__L.vi"() -> ("output_Solenoid_c__L"=w899:i32)  [unwired: 11 in]
      n512 = call "myRIO_BRig_RT_dataMTrig_Solenoid_Tcycle__L.vi"() -> ("output_Solenoid_Tcycle__L"=w910:i32)  [unwired: 11 in]
      n513 = call "myRIO_BRig_RT_dataMTrig_Solenoid_c__R.vi"() -> ("output_Solenoid_c__R"=w891:i32)  [unwired: 11 in]
      n514 = call "myRIO_BRig_RT_dataMTrig_Solenoid_Tcycle__R.vi"() -> ("output_Solenoid_Tcycle__R"=w894:i32)  [unwired: 11 in]
      n515 = call "myRIO_BRig_RT_dataMTrig_Audio_c__R.vi"() -> ("output_Audio_c__R"=w867:i32)  [unwired: 11 in]
      n516 = call "myRIO_BRig_RT_dataMTrig_Audio_Tcycle__R.vi"() -> ("output_Audio_Tcycle__R"=w873:i32)  [unwired: 11 in]
      n517 = call "myRIO_BRig_RT_dataMTrig_Laser_c.vi"() -> ("output_Laser_c"=w863:i32)  [unwired: 11 in]
      n518 = call "myRIO_BRig_RT_dataMTrig_Laser_Tcycle.vi"() -> ("output_Laser_Tcycle"=w872:i32)  [unwired: 11 in]
      n519 = Index Array(array=w904, index #1=w899, index #2=w910, index #3=w891, index #4=w894, index #5=w867, index #6=w873, index #7=w863, index #8=w872) -> (element #1=w909:u16, element #2=w908:u16, element #3=w893:u16, element #4=w892:u16, element #5=w871:u16, element #6=w870:u16, element #7=w869:u16, element #8=w868:u16)
      n520 = Add(x=w878, y=w909) -> (x+y=w906:u16)
      n521 = Add(x=w878, y=w893) -> (x+y=w897:u16)
      n522 = Add(x=w878, y=w871) -> (x+y=w885:u16)
      n523 = Add(x=w878, y=w869) -> (x+y=w881:u16)
      n524 = Less?(x=w906, y=w908) -> (x < y?=w874:bool)
      n525 = Less?(x=w897, y=w892) -> (x < y?=w875:bool)
      n526 = Less?(x=w885, y=w870) -> (x < y?=w876:bool)
      n527 = Less?(x=w881, y=w868) -> (x < y?=w877:bool)
      n528 = Decrement(x=w901) -> (x-1=w907:u16)
      n529 = Decrement(x=w895) -> (x-1=w898:u16)
      n530 = Decrement(x=w883) -> (x-1=w886:u16)
      n531 = Decrement(x=w879) -> (x-1=w882:u16)
      n532 = Select(t=w906, s=w874, f=u16 0) -> (s? t:f=w902:u16)
      n533 = Select(t=w901, s=w874, f=w907) -> (s? t:f=w903:u16)
      n534 = Select(t=w897, s=w875, f=u16 0) -> (s? t:f=w890:u16)
      n535 = Select(t=w895, s=w875, f=w898) -> (s? t:f=w888:u16)
      n536 = Select(t=w885, s=w876, f=u16 0) -> (s? t:f=w866:u16)
      n537 = Select(t=w883, s=w876, f=w886) -> (s? t:f=w864:u16)
      n538 = Select(t=w881, s=w877, f=u16 0) -> (s? t:f=w862:u16)
      n539 = Select(t=w879, s=w877, f=w882) -> (s? t:f=w860:u16)
      n540 = Replace Array Subset(array=w904, new element #1=w902, index #1=w899, new element #2=w903, index #2=w900, new element #3=w890, index #3=w891, new element #4=w888, index #4=w889, new element #5=w866, index #5=w867, new element #6=w864, index #6=w865, new element #7=w862, index #7=w863, new element #8=w860, index #8=w861) -> (w887:u16[])
    }
    frame 28 {
      # "Laser"
      # "Tcycle"
      # "count"
      # "Audio_R"
      # "Tcycle"
      # "count"
      # "Audio_L"
      # "Tcycle"
      # "count"
      n541 = call "myRIO_BRig_RT_dataMTrig_Audio_c__L.vi"() -> ("output_Audio_c__L"=w937:i32)  [unwired: 11 in]
      n542 = call "myRIO_BRig_RT_dataMTrig_Audio_Tcycle__L.vi"() -> ("output_Audio_Tcycle__L"=w943:i32)  [unwired: 11 in]
      n543 = call "myRIO_BRig_RT_dataMTrig_Audio_c__R.vi"() -> ("output_Audio_c__R"=w929:i32)  [unwired: 11 in]
      n544 = call "myRIO_BRig_RT_dataMTrig_Audio_Tcycle__R.vi"() -> ("output_Audio_Tcycle__R"=w930:i32)  [unwired: 11 in]
      n545 = call "myRIO_BRig_RT_dataMTrig_Laser_c.vi"() -> ("output_Laser_c"=w917:i32)  [unwired: 11 in]
      n546 = call "myRIO_BRig_RT_dataMTrig_Laser_Tcycle.vi"() -> ("output_Laser_Tcycle"=w920:i32)  [unwired: 11 in]
      n547 = Index Array(array=w949, index #1=w937, index #2=w943, index #3=w929, index #4=w930, index #5=w917, index #6=w920) -> (element #1=w942:u16, element #2=w941:u16, element #3=w932:u16, element #4=w931:u16, element #5=w919:u16, element #6=w918:u16)
      n548 = Add(x=w921, y=w942) -> (x+y=w946:u16)
      n549 = Add(x=w921, y=w932) -> (x+y=w935:u16)
      n550 = Add(x=w921, y=w919) -> (x+y=w924:u16)
      n551 = Less?(x=w946, y=w941) -> (x < y?=w911:bool)
      n552 = Less?(x=w935, y=w931) -> (x < y?=w912:bool)
      n553 = Less?(x=w924, y=w918) -> (x < y?=w913:bool)
      n554 = Decrement(x=w944) -> (x-1=w947:u16)
      n555 = Decrement(x=w933) -> (x-1=w936:u16)
      n556 = Decrement(x=w922) -> (x-1=w925:u16)
      n557 = Select(t=w946, s=w911, f=u16 0) -> (s? t:f=w940:u16)
      n558 = Select(t=w944, s=w911, f=w947) -> (s? t:f=w939:u16)
      n559 = Select(t=w935, s=w912, f=u16 0) -> (s? t:f=w927:u16)
      n560 = Select(t=w933, s=w912, f=w936) -> (s? t:f=w926:u16)
      n561 = Select(t=w924, s=w913, f=u16 0) -> (s? t:f=w915:u16)
      n562 = Select(t=w922, s=w913, f=w925) -> (s? t:f=w914:u16)
      n563 = Replace Array Subset(array=w949, new element #1=w940, index #1=w937, new element #2=w939, index #2=w938, new element #3=w927, index #3=w929, new element #4=w926, index #4=w928, new element #5=w915, index #5=w917, new element #6=w914, index #6=w916) -> (w948:u16[])
    }
    frame 29 {
      # "Laser"
      # "Tcycle"
      # "count"
      # "Audio_R"
      # "Tcycle"
      # "count"
      # "Audio_L"
      # "Tcycle"
      # "count"
      # "Solenoid__L"
      # "Tcycle"
      # "count"
      n564 = call "myRIO_BRig_RT_dataMTrig_Solenoid_c__L.vi"() -> ("output_Solenoid_c__L"=w953:i32)  [unwired: 11 in]
      n565 = call "myRIO_BRig_RT_dataMTrig_Solenoid_Tcycle__L.vi"() -> ("output_Solenoid_Tcycle__L"=w956:i32)  [unwired: 11 in]
      n566 = call "myRIO_BRig_RT_dataMTrig_Audio_c__L.vi"() -> ("output_Audio_c__L"=w984:i32)  [unwired: 11 in]
      n567 = call "myRIO_BRig_RT_dataMTrig_Audio_Tcycle__L.vi"() -> ("output_Audio_Tcycle__L"=w990:i32)  [unwired: 11 in]
      n568 = call "myRIO_BRig_RT_dataMTrig_Audio_c__R.vi"() -> ("output_Audio_c__R"=w976:i32)  [unwired: 11 in]
      n569 = call "myRIO_BRig_RT_dataMTrig_Audio_Tcycle__R.vi"() -> ("output_Audio_Tcycle__R"=w977:i32)  [unwired: 11 in]
      n570 = call "myRIO_BRig_RT_dataMTrig_Laser_c.vi"() -> ("output_Laser_c"=w964:i32)  [unwired: 11 in]
      n571 = call "myRIO_BRig_RT_dataMTrig_Laser_Tcycle.vi"() -> ("output_Laser_Tcycle"=w967:i32)  [unwired: 11 in]
      n572 = Index Array(array=w997, index #1=w953, index #2=w956, index #3=w984, index #4=w990, index #5=w976, index #6=w977, index #7=w964, index #8=w967) -> (element #1=w955:u16, element #2=w954:u16, element #3=w989:u16, element #4=w988:u16, element #5=w979:u16, element #6=w978:u16, element #7=w966:u16, element #8=w965:u16)
      n573 = Add(x=w968, y=w955) -> (x+y=w999:u16)
      n574 = Add(x=w968, y=w989) -> (x+y=w993:u16)
      n575 = Add(x=w968, y=w979) -> (x+y=w982:u16)
      n576 = Add(x=w968, y=w966) -> (x+y=w971:u16)
      n577 = Less?(x=w999, y=w954) -> (x < y?=w957:bool)
      n578 = Less?(x=w993, y=w988) -> (x < y?=w958:bool)
      n579 = Less?(x=w982, y=w978) -> (x < y?=w959:bool)
      n580 = Less?(x=w971, y=w965) -> (x < y?=w960:bool)
      n581 = Decrement(x=w996) -> (x-1=w1000:u16)
      n582 = Decrement(x=w991) -> (x-1=w994:u16)
      n583 = Decrement(x=w980) -> (x-1=w983:u16)
      n584 = Decrement(x=w969) -> (x-1=w972:u16)
      n585 = Select(t=w999, s=w957, f=u16 0) -> (s? t:f=w952:u16)
      n586 = Select(t=w996, s=w957, f=w1000) -> (s? t:f=w950:u16)
      n587 = Select(t=w993, s=w958, f=u16 0) -> (s? t:f=w987:u16)
      n588 = Select(t=w991, s=w958, f=w994) -> (s? t:f=w986:u16)
      n589 = Select(t=w982, s=w959, f=u16 0) -> (s? t:f=w974:u16)
      n590 = Select(t=w980, s=w959, f=w983) -> (s? t:f=w973:u16)
      n591 = Select(t=w971, s=w960, f=u16 0) -> (s? t:f=w962:u16)
      n592 = Select(t=w969, s=w960, f=w972) -> (s? t:f=w961:u16)
      n593 = Replace Array Subset(array=w997, new element #1=w952, index #1=w953, new element #2=w950, index #2=w951, new element #3=w987, index #3=w984, new element #4=w986, index #4=w985, new element #5=w974, index #5=w976, new element #6=w973, index #6=w975, new element #7=w962, index #7=w964, new element #8=w961, index #8=w963) -> (w995:u16[])
    }
    frame 30 {
      # "Laser"
      # "Tcycle"
      # "count"
      # "Audio_R"
      # "Tcycle"
      # "count"
      # "Audio_L"
      # "Tcycle"
      # "count"
      # "Solenoid__R"
      # "Tcycle"
      # "count"
      n594 = call "myRIO_BRig_RT_dataMTrig_Solenoid_c__R.vi"() -> ("output_Solenoid_c__R"=w1043:i32)  [unwired: 11 in]
      n595 = call "myRIO_BRig_RT_dataMTrig_Solenoid_Tcycle__R.vi"() -> ("output_Solenoid_Tcycle__R"=w1046:i32)  [unwired: 11 in]
      n596 = call "myRIO_BRig_RT_dataMTrig_Audio_c__L.vi"() -> ("output_Audio_c__L"=w1028:i32)  [unwired: 11 in]
      n597 = call "myRIO_BRig_RT_dataMTrig_Audio_Tcycle__L.vi"() -> ("output_Audio_Tcycle__L"=w1034:i32)  [unwired: 11 in]
      n598 = call "myRIO_BRig_RT_dataMTrig_Audio_c__R.vi"() -> ("output_Audio_c__R"=w1020:i32)  [unwired: 11 in]
      n599 = call "myRIO_BRig_RT_dataMTrig_Audio_Tcycle__R.vi"() -> ("output_Audio_Tcycle__R"=w1021:i32)  [unwired: 11 in]
      n600 = call "myRIO_BRig_RT_dataMTrig_Laser_c.vi"() -> ("output_Laser_c"=w1008:i32)  [unwired: 11 in]
      n601 = call "myRIO_BRig_RT_dataMTrig_Laser_Tcycle.vi"() -> ("output_Laser_Tcycle"=w1011:i32)  [unwired: 11 in]
      n602 = Index Array(array=w1051, index #1=w1043, index #2=w1046, index #3=w1028, index #4=w1034, index #5=w1020, index #6=w1021, index #7=w1008, index #8=w1011) -> (element #1=w1045:u16, element #2=w1044:u16, element #3=w1033:u16, element #4=w1032:u16, element #5=w1023:u16, element #6=w1022:u16, element #7=w1010:u16, element #8=w1009:u16)
      n603 = Add(x=w1012, y=w1045) -> (x+y=w1049:u16)
      n604 = Add(x=w1012, y=w1033) -> (x+y=w1037:u16)
      n605 = Add(x=w1012, y=w1023) -> (x+y=w1026:u16)
      n606 = Add(x=w1012, y=w1010) -> (x+y=w1015:u16)
      n607 = Less?(x=w1049, y=w1044) -> (x < y?=w1001:bool)
      n608 = Less?(x=w1037, y=w1032) -> (x < y?=w1002:bool)
      n609 = Less?(x=w1026, y=w1022) -> (x < y?=w1003:bool)
      n610 = Less?(x=w1015, y=w1009) -> (x < y?=w1004:bool)
      n611 = Decrement(x=w1047) -> (x-1=w1050:u16)
      n612 = Decrement(x=w1035) -> (x-1=w1038:u16)
      n613 = Decrement(x=w1024) -> (x-1=w1027:u16)
      n614 = Decrement(x=w1013) -> (x-1=w1016:u16)
      n615 = Select(t=w1049, s=w1001, f=u16 0) -> (s? t:f=w1042:u16)
      n616 = Select(t=w1047, s=w1001, f=w1050) -> (s? t:f=w1040:u16)
      n617 = Select(t=w1037, s=w1002, f=u16 0) -> (s? t:f=w1031:u16)
      n618 = Select(t=w1035, s=w1002, f=w1038) -> (s? t:f=w1030:u16)
      n619 = Select(t=w1026, s=w1003, f=u16 0) -> (s? t:f=w1018:u16)
      n620 = Select(t=w1024, s=w1003, f=w1027) -> (s? t:f=w1017:u16)
      n621 = Select(t=w1015, s=w1004, f=u16 0) -> (s? t:f=w1006:u16)
      n622 = Select(t=w1013, s=w1004, f=w1016) -> (s? t:f=w1005:u16)
      n623 = Replace Array Subset(array=w1051, new element #1=w1042, index #1=w1043, new element #2=w1040, index #2=w1041, new element #3=w1031, index #3=w1028, new element #4=w1030, index #4=w1029, new element #5=w1018, index #5=w1020, new element #6=w1017, index #6=w1019, new element #7=w1006, index #7=w1008, new element #8=w1005, index #8=w1007) -> (w1039:u16[])
    }
    frame 31 {
      # "Laser"
      # "Tcycle"
      # "count"
      # "Audio_R"
      # "Tcycle"
      # "count"
      # "Audio_L"
      # "Tcycle"
      # "count"
      # "Solenoid__R"
      # "Tcycle"
      # "count"
      # "Solenoid__L"
      # "Tcycle"
      # "count"
      n624 = call "myRIO_BRig_RT_dataMTrig_Solenoid_c__L.vi"() -> ("output_Solenoid_c__L"=w1103:i32)  [unwired: 11 in]
      n625 = call "myRIO_BRig_RT_dataMTrig_Solenoid_Tcycle__L.vi"() -> ("output_Solenoid_Tcycle__L"=w1114:i32)  [unwired: 11 in]
      n626 = call "myRIO_BRig_RT_dataMTrig_Solenoid_c__R.vi"() -> ("output_Solenoid_c__R"=w1095:i32)  [unwired: 11 in]
      n627 = call "myRIO_BRig_RT_dataMTrig_Solenoid_Tcycle__R.vi"() -> ("output_Solenoid_Tcycle__R"=w1098:i32)  [unwired: 11 in]
      n628 = call "myRIO_BRig_RT_dataMTrig_Audio_c__L.vi"() -> ("output_Audio_c__L"=w1080:i32)  [unwired: 11 in]
      n629 = call "myRIO_BRig_RT_dataMTrig_Audio_Tcycle__L.vi"() -> ("output_Audio_Tcycle__L"=w1086:i32)  [unwired: 11 in]
      n630 = call "myRIO_BRig_RT_dataMTrig_Audio_c__R.vi"() -> ("output_Audio_c__R"=w1072:i32)  [unwired: 11 in]
      n631 = call "myRIO_BRig_RT_dataMTrig_Audio_Tcycle__R.vi"() -> ("output_Audio_Tcycle__R"=w1073:i32)  [unwired: 11 in]
      n632 = call "myRIO_BRig_RT_dataMTrig_Laser_c.vi"() -> ("output_Laser_c"=w1060:i32)  [unwired: 11 in]
      n633 = call "myRIO_BRig_RT_dataMTrig_Laser_Tcycle.vi"() -> ("output_Laser_Tcycle"=w1063:i32)  [unwired: 11 in]
      n634 = Index Array(array=w1108, index #1=w1103, index #2=w1114, index #3=w1095, index #4=w1098, index #5=w1080, index #6=w1086, index #7=w1072, index #8=w1073, index #9=w1060, index #10=w1063) -> (element #1=w1113:u16, element #2=w1112:u16, element #3=w1097:u16, element #4=w1096:u16, element #5=w1085:u16, element #6=w1084:u16, element #7=w1075:u16, element #8=w1074:u16, element #9=w1062:u16, element #10=w1061:u16)
      n635 = Add(x=w1064, y=w1113) -> (x+y=w1110:u16)
      n636 = Add(x=w1064, y=w1097) -> (x+y=w1101:u16)
      n637 = Add(x=w1064, y=w1085) -> (x+y=w1089:u16)
      n638 = Add(x=w1064, y=w1075) -> (x+y=w1078:u16)
      n639 = Add(x=w1064, y=w1062) -> (x+y=w1067:u16)
      n640 = Less?(x=w1110, y=w1112) -> (x < y?=w1052:bool)
      n641 = Less?(x=w1101, y=w1096) -> (x < y?=w1053:bool)
      n642 = Less?(x=w1089, y=w1084) -> (x < y?=w1054:bool)
      n643 = Less?(x=w1078, y=w1074) -> (x < y?=w1055:bool)
      n644 = Less?(x=w1067, y=w1061) -> (x < y?=w1056:bool)
      n645 = Decrement(x=w1105) -> (x-1=w1111:u16)
      n646 = Decrement(x=w1099) -> (x-1=w1102:u16)
      n647 = Decrement(x=w1087) -> (x-1=w1090:u16)
      n648 = Decrement(x=w1076) -> (x-1=w1079:u16)
      n649 = Decrement(x=w1065) -> (x-1=w1068:u16)
      n650 = Select(t=w1110, s=w1052, f=u16 0) -> (s? t:f=w1106:u16)
      n651 = Select(t=w1105, s=w1052, f=w1111) -> (s? t:f=w1107:u16)
      n652 = Select(t=w1101, s=w1053, f=u16 0) -> (s? t:f=w1094:u16)
      n653 = Select(t=w1099, s=w1053, f=w1102) -> (s? t:f=w1092:u16)
      n654 = Select(t=w1089, s=w1054, f=u16 0) -> (s? t:f=w1083:u16)
      n655 = Select(t=w1087, s=w1054, f=w1090) -> (s? t:f=w1082:u16)
      n656 = Select(t=w1078, s=w1055, f=u16 0) -> (s? t:f=w1070:u16)
      n657 = Select(t=w1076, s=w1055, f=w1079) -> (s? t:f=w1069:u16)
      n658 = Select(t=w1067, s=w1056, f=u16 0) -> (s? t:f=w1058:u16)
      n659 = Select(t=w1065, s=w1056, f=w1068) -> (s? t:f=w1057:u16)
      n660 = Replace Array Subset(array=w1108, new element #1=w1106, index #1=w1103, new element #2=w1107, index #2=w1104, new element #3=w1094, index #3=w1095, new element #4=w1092, index #4=w1093, new element #5=w1083, index #5=w1080, new element #6=w1082, index #6=w1081, new element #7=w1070, index #7=w1072, new element #8=w1069, index #8=w1071, new element #9=w1058, index #9=w1060, new element #10=w1057, index #10=w1059) -> (w1091:u16[])
    }
  }
  "output_dataMTrig" <- w18
  "output_Solenoid_L" <- w14
  "output_Solenoid_R" <- w13
  "output_Audio_L" <- w12
  "output_Audio_R" <- w11
  "output_Laser" <- w10
